vi "Actor Core.vi"(8 "error in":errorcluster, 11 "Data Viewer in":refnum<class "NI Force Task.lvclass">) -> (0 "error out":errorcluster, 3 "Actor out":refnum<class "Actor.lvclass">)   [LabVIEW 2020, in "NI Force Task.lvlib" / "NI Force Task.lvclass"]
doc: "The user interface for this panel.\n----\nCopyright: MGI 2016\nAuthor: Derek Trepanier"
uses:
  NI Force Task.lvclass
  C:/Program Files/National Instruments/LabVIEW 2020/vi.lib/MGI/Panel Manager/Panel Actor/Panel Actor/Panel Actor.lvclass
  C:/Program Files/National Instruments/LabVIEW 2020/vi.lib/ActorFramework/Actor/Actor.lvclass
  <vilib>/ActorFramework/Actor/Actor.lvclass
  Task info df.ctl
  NI Force Task.lvclass/NI Force Task.ctl
  <vilib>/ActorFramework/Actor/Actor.lvclass/Actor.ctl
  <vilib>/ActorFramework/Message Enqueuer/Message Enqueuer.lvclass/Message Enqueuer.ctl
  GUI Interface Messages/MVC Collection Finished Msg/MVC Collection Finished Msg.lvclass/MVC Collection Finished Msg.ctl
  GUI Interface Messages/Force Calibration Finished Msg/Force Calibration Finished Msg.lvclass/Force Calibration Finished Msg.ctl
  GUI Interface Messages/Pot Calibration Finished Msg/Pot Calibration Finished Msg.lvclass/Pot Calibration Finished Msg.ctl
  NI Force Task Messages/Update Template Graph Msg/Update Template Graph Msg.lvclass/Update Template Graph Msg.ctl
  GUI/NI Tasl df.ctl
  Movement Template df.ctl
  <vilib>/Utility/miscctls.llb/LVBoundsTypeDef.ctl
  <vilib>/DAQmx/read.llb/DAQmx Read (Analog 1D Wfm NChan 1Samp).vi
  <vilib>/Analysis/baseanly.llb/Mean (DBL).vi
  <vilib>/ActorFramework/Message Enqueuer/Init from Existing Queue.vi
  <vilib>/ActorFramework/Message Enqueuer/Enqueue.vi
  GUI Interface Messages/MVC Collection Finished Msg/MVC Collection Finished Msg.lvclass
  C:/Program Files/National Instruments/LabVIEW 2020/vi.lib/ActorFramework/Message/Message.lvclass
  GUI Interface Messages/Force Calibration Finished Msg/Force Calibration Finished Msg.lvclass
  GUI Interface Messages/Pot Calibration Finished Msg/Pot Calibration Finished Msg.lvclass
  NI Force Task Messages/Update Template Graph Msg/Update Template Graph Msg.lvclass
  <vilib>/ActorFramework/Stop Msg/Stop Msg.lvclass
  GUI Interface Messages/Task Panel Closed Msg/Task Panel Closed Msg.lvclass
  <vilib>/Waveform/WDTOps.llb/WDT Get Waveform Time Array DBL.vi
  <vilib>/DAQmx/miscellaneous.llb/DAQmx Fill In Error Info.vi
  <vilib>/Analysis/2dsp.llb/Decimate (continuous, DBL).vi
  <vilib>/ActorFramework/Message Priority Queue/Priority Enqueue.vi
  <vilib>/ActorFramework/Message Enqueuer/Message Enqueuer.lvclass
  <vilib>/MGI/Panel Manager/Panel Actor/Panel Actor/Panel Actor.lvclass
  NI Force Task Messages/Process Live Data Q Msg/Process Live Data Q Msg.lvclass
  <vilib>/Analysis/NI_AALBase.lvlib
  <vilib>/Analysis/NI_AALPro.lvlib
  NI Force Task Messages/Process Live Data Q Mov Msg/Process Live Data Q Mov Msg.lvclass
  NI Force Task Messages/Stop Trial Msg/Stop Trial Msg.lvclass
  NI Force Task Messages/End Scanning Trial Msg/End Scanning Trial Msg.lvclass
  NI Force Task Messages/Process Live Data Q EMG Msg/Process Live Data Q EMG Msg.lvclass
panel:
  out "Countdown":string
  in  "EMG Only?":bool
  out "Task Info Backup":T1={"Number of Trials"=1, "Sampling Rate (Hz)"=200, "Trial Duration (s)"=10, "Adjusted MVC (N)"=5.0, "R Phase"=0, "L Phase"=0, "L Pattern"=1, "R Pattern"=1, "Time Between Trials (s)"=5, "Lissajous Speed"=200} {"Lissajous Speed" min=1 max=200; "Time Between Trials (s)" min=1 step=1; "R Pattern" min=1 max=20 step=1; "L Pattern" min=1 max=20 step=1; "L Phase" max=360 step=1; "R Phase" max=360 step=1; "Adjusted MVC (N)" min=1.0 step=1.0; "Trial Duration (s)" min=1 step=1; "Sampling Rate (Hz)" min=1 step=1; "Number of Trials" min=1 step=1}
  in  "Scanning Task?":bool
  in  "Wait":bool
  out "Task Info In":T1={"Number of Trials"=1, "Sampling Rate (Hz)"=200, "Trial Duration (s)"=10, "Adjusted MVC (N)"=5.0, "R Phase"=0, "L Phase"=0, "L Pattern"=1, "R Pattern"=1, "Time Between Trials (s)"=5, "Lissajous Speed"=200} {"Lissajous Speed" min=1 max=200; "Time Between Trials (s)" min=1 step=1; "R Pattern" min=1 max=20 step=1; "L Pattern" min=1 max=20 step=1; "L Phase" max=360 step=1; "R Phase" max=360 step=1; "Adjusted MVC (N)" min=1.0 step=1.0; "Trial Duration (s)" min=1 step=1; "Sampling Rate (Hz)" min=1 step=1; "Number of Trials" min=1 step=1}
  in  "Movement?":bool
  in  "Decimation factor":i32=1
  out "Acquire EMG":bool
  in  "Rate Hz":u16
  out "Live Data":cluster{"Result":dbl[], "Result":dbl[]}(graph)
  in  "Force Calibration Cluster":cluster{"Left":dbl, "Right":dbl}
  in  "Chnl Names":string[](array[string])
  in  "TDMS File Ref":refnum<k34>
  in  "Task Ref":refnum<k21>
  in  "Trial Num":i32
  in  "Stop Acquire":bool
  out "Template Graph":cluster{"Result":dbl[], "Result":dbl[]}(graph)
  # "Right Arm"
  # "Left Arm"
  # "Right Arm"
  # "Left Arm"
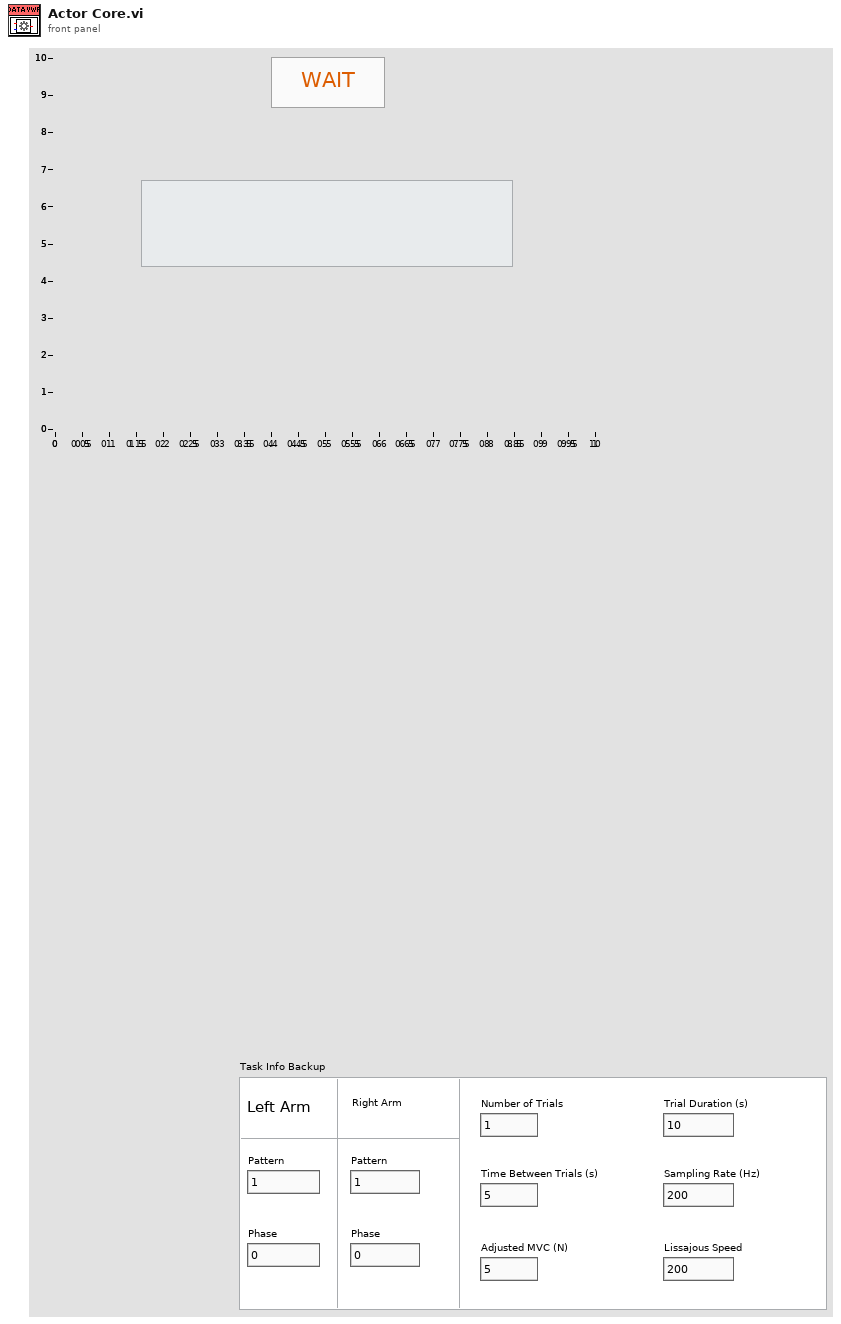
[diagram p1: front panel]
types:
  T1 = typedef "Task info df.ctl" = cluster{"Number of Trials":u8, "Sampling Rate (Hz)":u16, "Trial Duration (s)":u8, "Adjusted MVC (N)":dbl, "R Phase":i32, "L Phase":i32, "L Pattern":u8, "R Pattern":u8, "Time Between Trials (s)":u8, "Lissajous Speed":u16}
  T2 = cluster{"Template Data Update":refnum<user-event>, "Trial Number Update":refnum<user-event>, "Stop Acquire":refnum<user-event>, "Shut Down":refnum<user-event>, "Update Task Plot":refnum<user-event>, "Calibrate Force":refnum<user-event>, "Collect MVC":refnum<user-event>, "Acquire EMG":refnum<user-event>, "Movement? Update":refnum<user-event>, "Calibrate Pot":refnum<user-event>, "Scanning Task?":refnum<user-event>, "EMG only?":refnum<user-event>, "Countdown update":refnum<user-event>}
  T3 = cluster{"Event Registration Refnum":refnum<event-registration>, "Pnl Actor":refnum<event-registration>}
  T4 = typedef "Movement Template df.ctl" = enum16{"Idle", "Update Scanning Template", "Close Helper Loop", "Countdown"}
  T5 = typedef "NI Tasl df.ctl" = enum16{"Idle", "Acquire Force", "Acquire Force and EMG", "Acquire Movement", "Acquire Movement and EMG", "Calibrate Force", "Calibrate Potentiometers", "Collect MVC", "Close Helper Loop", "Collect EMG only", "Countdown"}
  T6 = typedef "LVRectTypeDef.ctl" = cluster{"Left":i16, "Top":i16, "Right":i16, "Bottom":i16}
  T7 = typedef "LVBoundsTypeDef.ctl" = cluster{"Width":u32, "Height":u32}
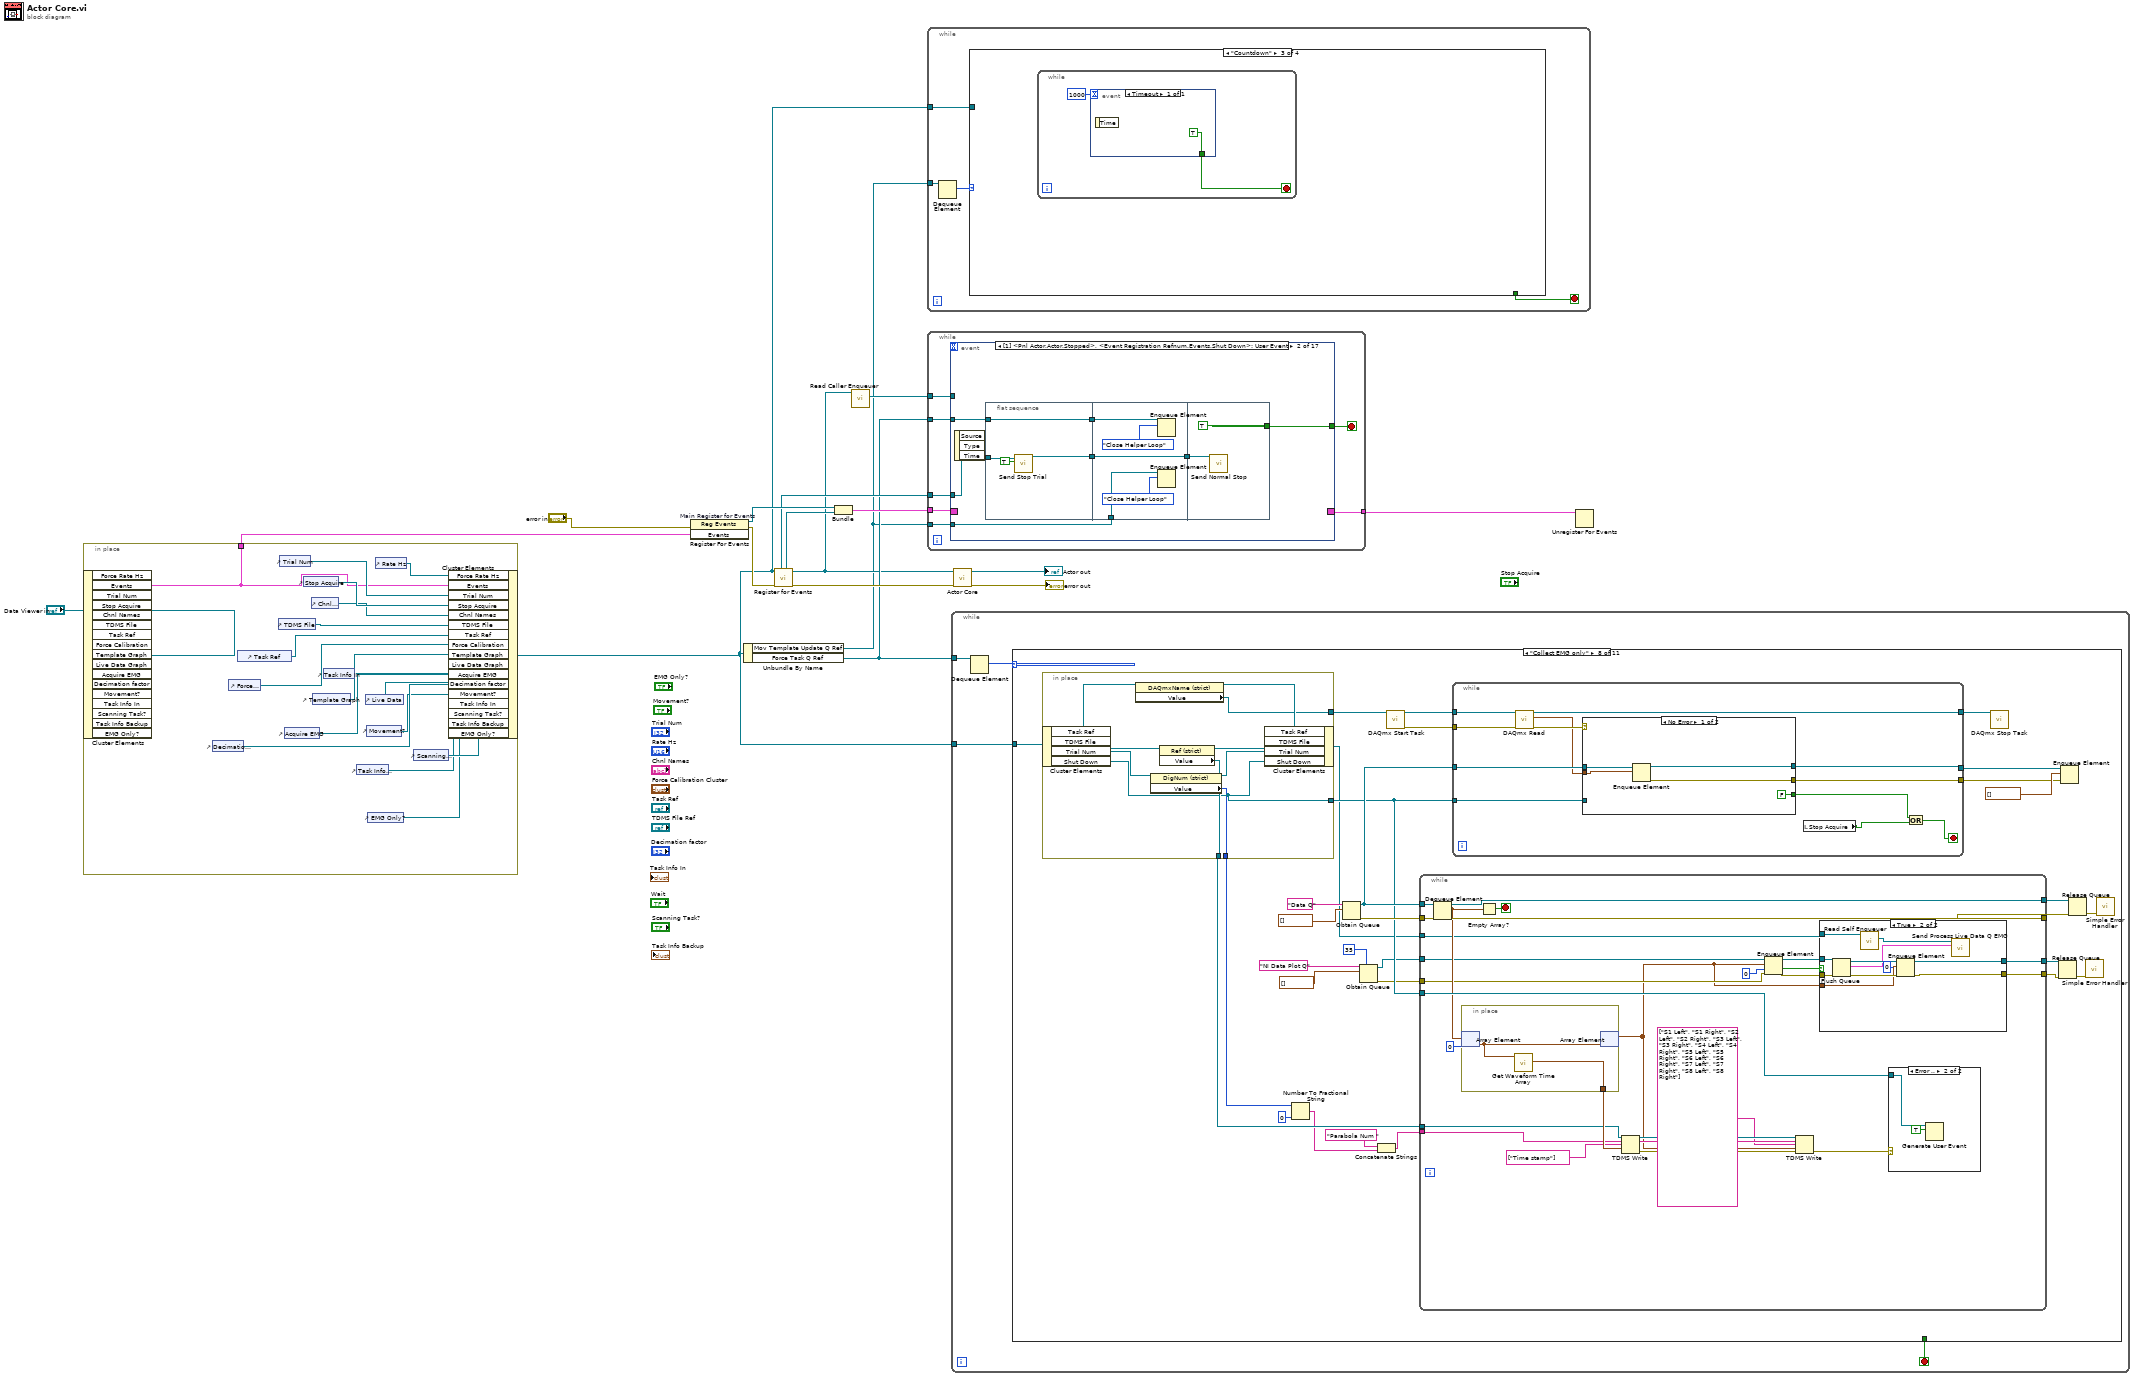
[diagram p0: block diagram]
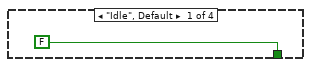
[diagram p2: hidden frame]
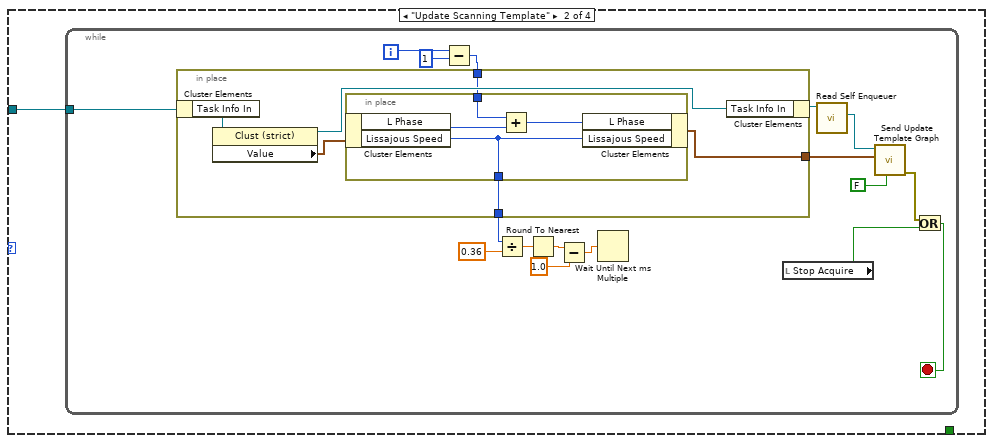
[diagram p3: hidden frame]
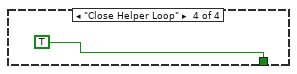
[diagram p4: hidden frame]
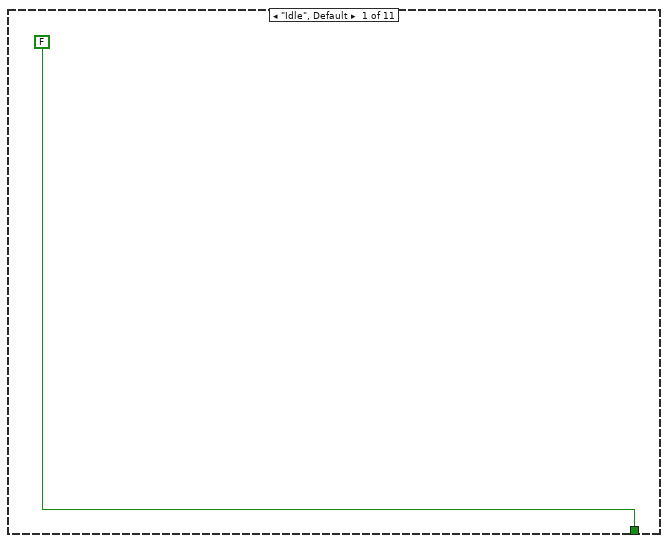
[diagram p5: hidden frame]
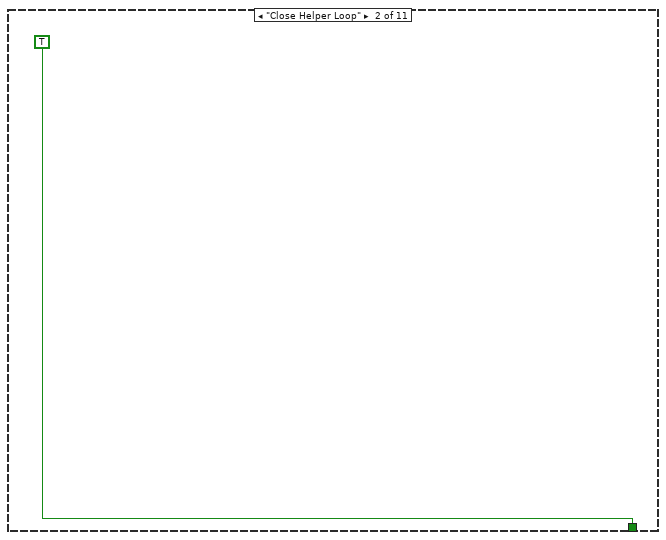
[diagram p6: hidden frame]
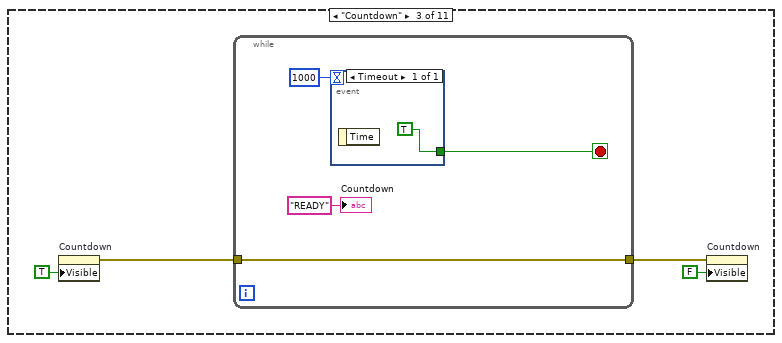
[diagram p7: hidden frame]
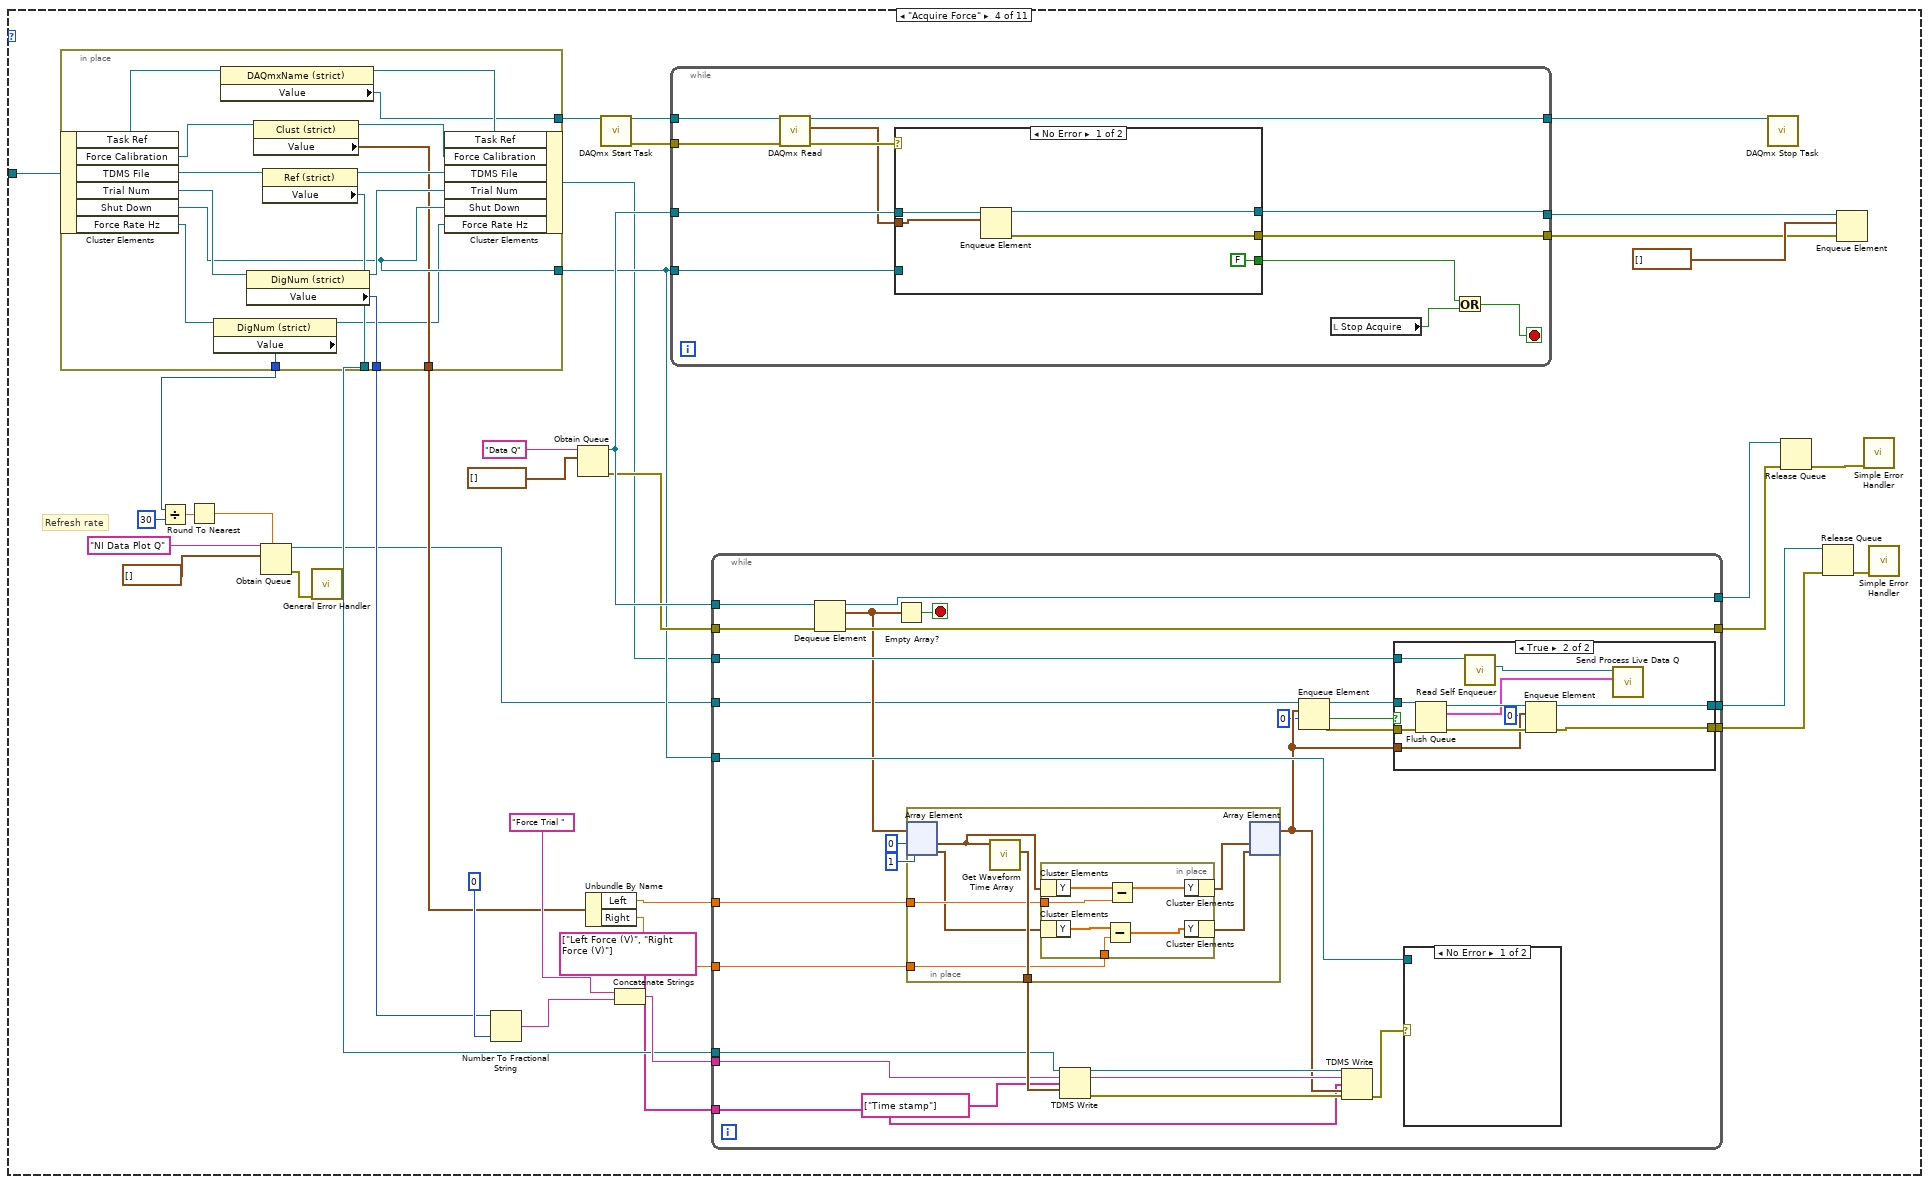
[diagram p8: hidden frame]
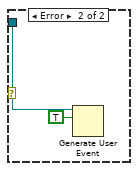
[diagram p10: hidden frame]
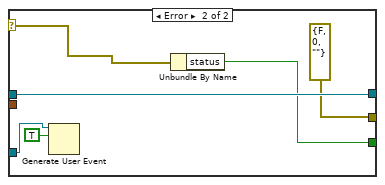
[diagram p11: hidden frame]
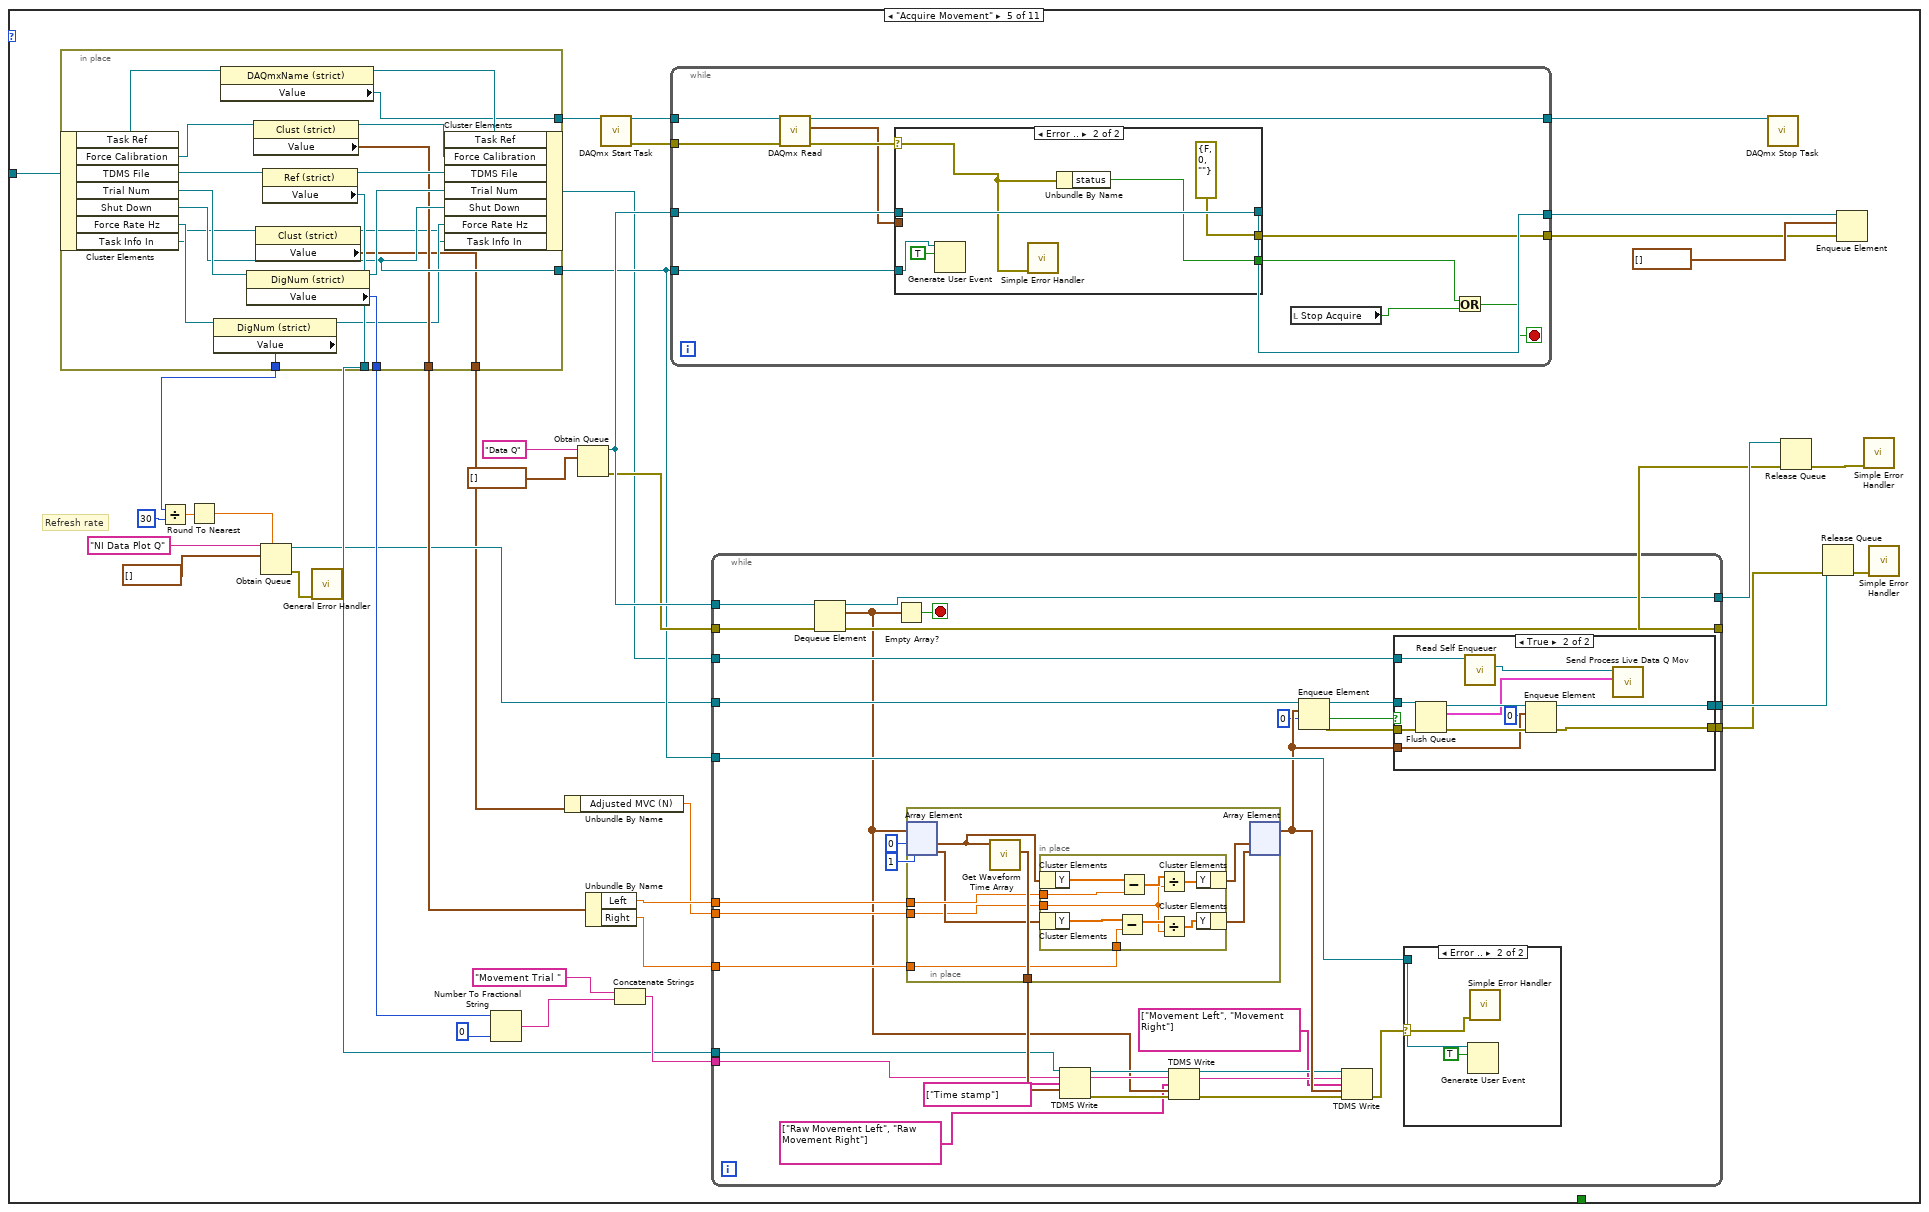
[diagram p12: hidden frame]
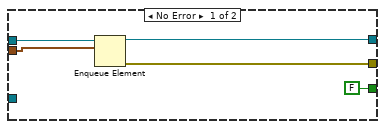
[diagram p15: hidden frame]
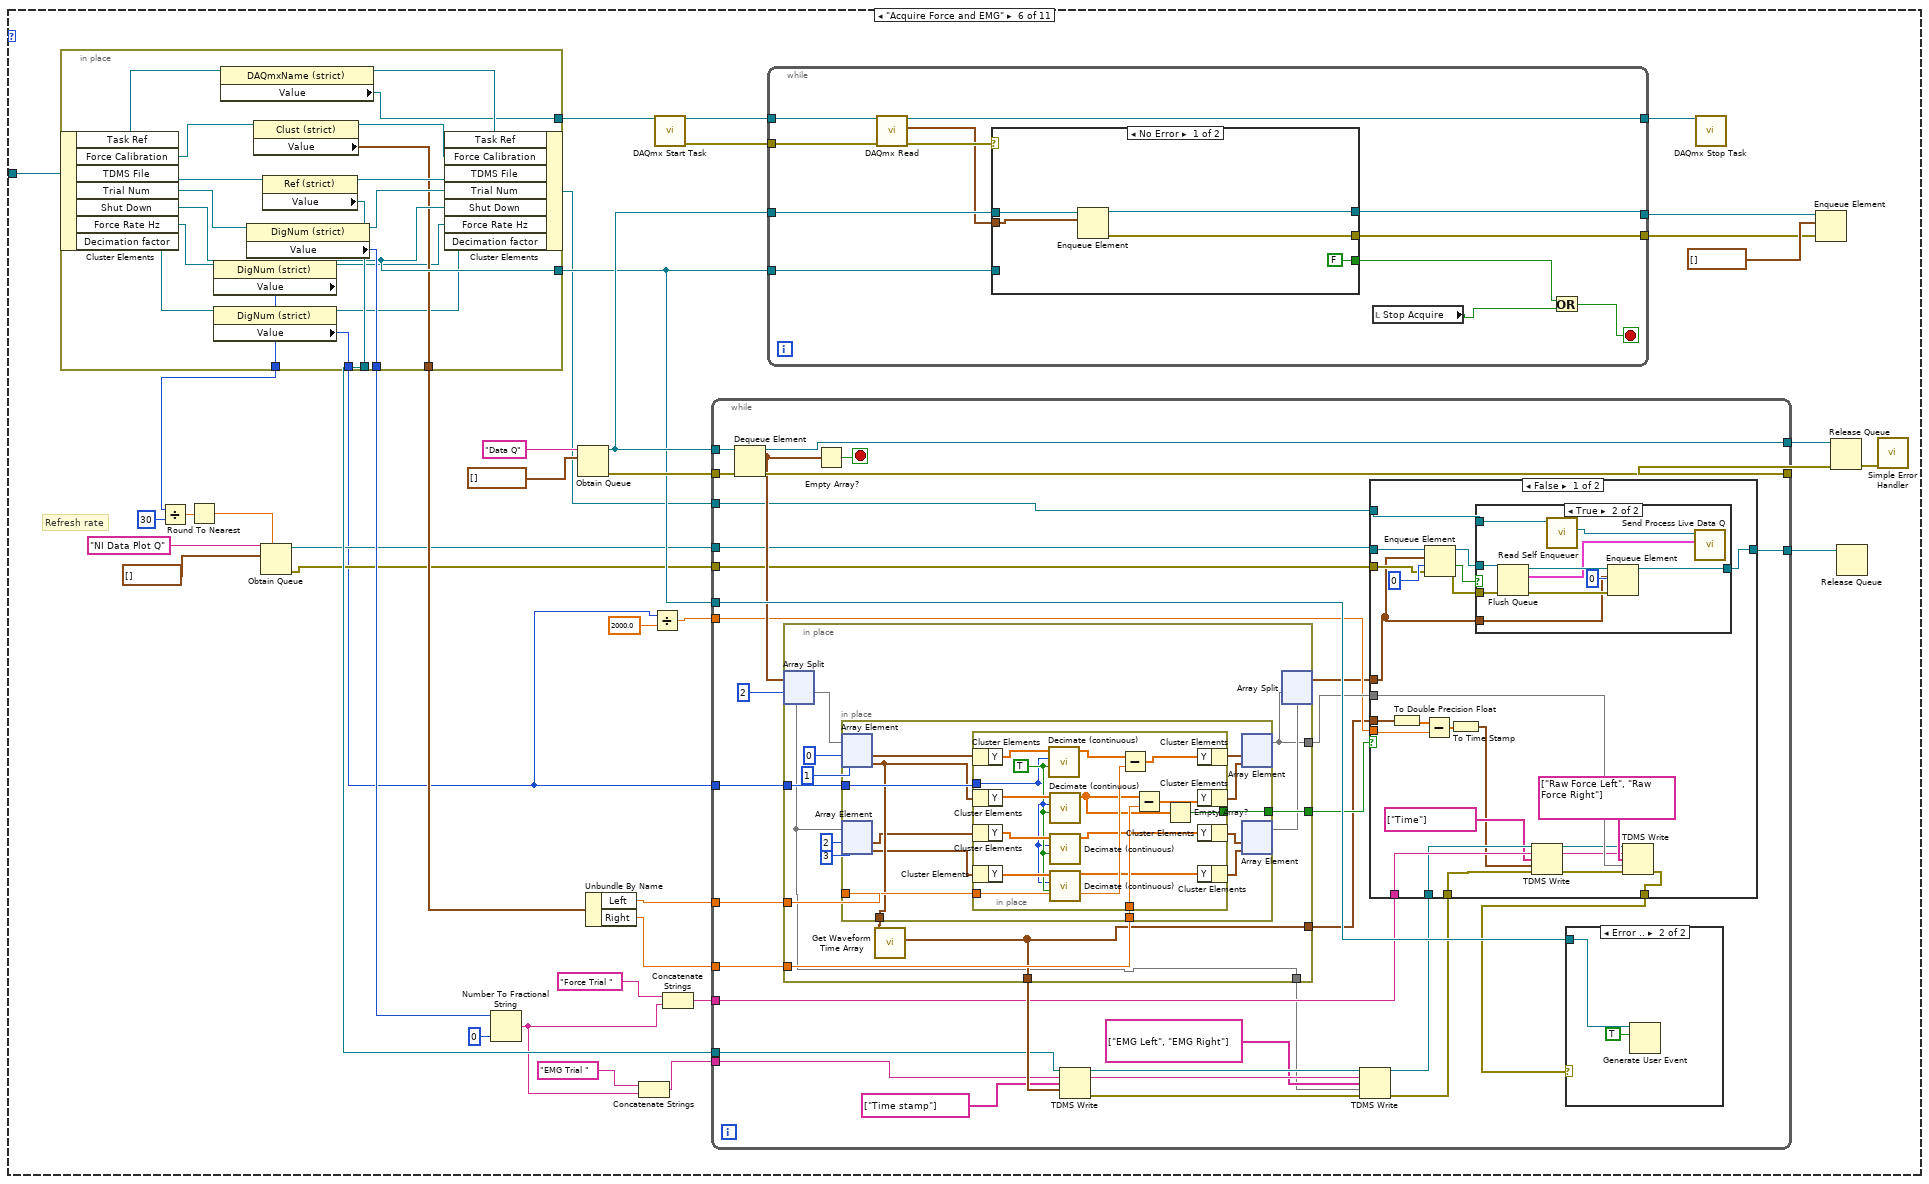
[diagram p16: hidden frame]
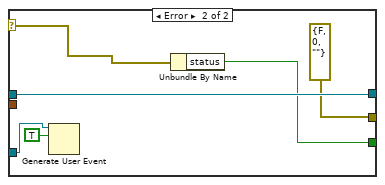
[diagram p20: hidden frame]
diagram:
  n1 = in-place {
    in-place-border: [w28] -> w6
    n2 = in-place-cluster #1("Data Viewer in") -> ("Events"=w28:T2)  [unwired: 16 out]
    n3 = control-ref of="Decimation factor"() -> (w23:refnum<vi>)
    n4 = control-ref of="Force Calibration Cluster"() -> (w29:refnum<vi>)
    n5 = control-ref of="Task Ref"() -> (w31:refnum<vi>)
    n6 = control-ref of="TDMS File"() -> (w30:refnum<vi>)
    n7 = control-ref of="Trial Num"() -> (w34:refnum<vi>)
    n8 = control-ref of="Acquire EMG"() -> (w24:refnum<vi>)
    n9 = control-ref of="Stop Acquire"() -> (w33:refnum<vi>)
    n10 = control-ref of="Chnl Names"() -> (w32:refnum<vi>)
    n11 = control-ref of="Template Graph"() -> (w27:refnum<vi>)
    n12 = control-ref of="Task Info In"() -> (w21:refnum<vi>)
    n13 = control-ref of="Task Info Backup"() -> (w19:refnum<vi>)
    n14 = control-ref of="Live Data"() -> (w26:refnum<vi>)
    n15 = control-ref of="Movement?"() -> (w22:refnum<vi>)
    n16 = control-ref of="EMG Only?"() -> (w18:refnum<vi>)
    n17 = control-ref of="Rate Hz"() -> (w25:refnum<vi>)
    n18 = control-ref of="Scanning Task?"() -> (w20:refnum<vi>)
    n19 = in-place-cluster #1("Force Rate Hz"=w25, "Events"=w28, "Trial Num"=w34, "Stop Acquire"=w33, "Chnl Names"=w32, "TDMS File"=w30, "Task Ref"=w31, "Force Calibration"=w29, "Template Graph"=w27, "Live Data Graph"=w26, "Acquire EMG"=w24, "Decimation factor"=w23, "Movement?"=w22, "Task Info In"=w21, "Scanning Task?"=w20, "Task Info Backup"=w19, "EMG Only?"=w18) -> (w1:refnum<class "NI Force Task.lvclass">)
  }
  n20 = register-events "Main Register for Events"(error in="error in", w6) -> (reference out=w12:refnum<event-registration>, error out=w13:errorcluster)  [unwired: 1 in]
  n21 = Unbundle By Name(w1) -> ("Mov Template Update Q Ref"=w2:refnum<queue>, "Force Task Q Ref"=w5:refnum<queue>)
  n22 = call <vilib>:"Register for Events.vi"("Error In"=w13, "Panel Actor in"=w1) -> ("Error Out"=w15:errorcluster, "Panel Actor out"=w4:refnum<class "NI Force Task.lvclass">, "Pnl Actor"=w11:refnum<event-registration>, "Self Enqueuer"=w7:refnum<class "Message Enqueuer.lvclass">)  [unwired: 6 in]
  n23 = Bundle("Event Registration Refnum"=w12, "Pnl Actor"=w11) -> (w10:T3)  [unwired: 1 in]
  n24 = call <vilib>:"Read Caller Enqueuer.vi"("Actor"=w4) -> ("Caller Enqueuer"=w3:refnum<class "Message Enqueuer.lvclass">)  [unwired: 10 in]
  n25 = while {
    tunnel: w2 -> [w38]
    tunnel: w1 -> [w35]
    stop <- w36 stop-if-true
    n26 = Dequeue Element(queue=w38) -> (element=w37:T4)  [unwired: 2 in, 3 out]
    n27 = case shown="\"Countdown\"" w37 {
      tunnel: [FALSE _ _ TRUE] -> w36
      tunnel: w35 -> [_ w40 _ _]
      frame "Idle", Default {
      }
      frame "Update Scanning Template" {
        n28 = while {
          tunnel: w40 -> [w41]
          i -> [w48]
          stop <- w49 stop-if-true
          n29 = Subtract(x=w48, y=1) -> (x-y=w47:i32)
          n30 = in-place {
            in-place-border: [w60] -> w55
            in-place-border: [w59] -> w52
            in-place-border: w47 -> [w58]
            n31 = in-place-cluster #2(w41) -> ("Task Info In"=w63:refnum<vi>)
            n32 = property class="Clust (strict)"(reference=w63) -> (reference out=w61:refnum<vi>, "Value"=w62:T1)  [unwired: 1 in, 1 out]
            n33 = in-place {
              in-place-border: [w67] -> w60
              in-place-border: w58 -> [w64]
              n34 = in-place-cluster #3(w62) -> ("L Phase"=w66:i32, "Lissajous Speed"=w67:u16)
              n35 = Add(x=w64, y=w66) -> (x+y=w65:i32)
              n36 = in-place-cluster #3("L Phase"=w65, "Lissajous Speed"=w67) -> (w59:T1)
            }
            n37 = in-place-cluster #2("Task Info In"=w61) -> (w54:refnum<class "NI Force Task.lvclass">)
          }
          n38 = Divide(x=w55, y=0.36) -> (x/y=w57:dbl)
          n39 = Round To Nearest(number=w57) -> (nearest integer value=w44:dbl)
          n40 = Subtract(x=w44, y=1.0) -> (x-y=w45:dbl)
          n41 = Wait Until Next ms Multiple(millisecond multiple=w45) -> ()  [unwired: 1 out]
          n42 = local read "Stop Acquire"() -> (w50:bool)
          n43 = call <vilib>:"Read Self Enqueuer.vi"("Actor"=w54) -> ("Self Enqueuer"=w53:refnum<class "Message Enqueuer.lvclass">)  [unwired: 10 in]
          n44 = call "Send Update Template Graph.vi"("Set Task Info?"=FALSE, "Task Info In"=w52, "Message Enqueuer in"=w53) -> ("error out"=w51:errorcluster)  [unwired: 7 in, 1 out]
          n45 = Or(x=w51, y=w50) -> (x .or. y?=w49:bool)
        }
      }
      frame "Countdown" {
        n46 = while {
          stop <- w68 stop-if-true
          n47 = event shown="[0] Timeout" {
            selector: _ -> [_]
            dyn-events: _ -> [_]
            timeout: 1000 -> [_]
            tunnel: [TRUE] -> w68
            event Timeout {
              n48 = event-data() -> ()  [unwired: 1 in, 1 out]
            }
          }
        }
      }
      frame "Close Helper Loop" {
      }
    }
  }
  n49 = while {
    tunnel: w7 -> [w77]
    tunnel: w10 -> [w76]
    tunnel: [w75] -> w9
    tunnel: w5 -> [w74]
    tunnel: w3 -> [w73]
    tunnel: w2 -> [w72]
    stop <- w78 stop-if-true
    n50 = event shown="[1] <Pnl Actor.Actor.Stopped>, <Event Registration Refnum.Events.Shut Down>: User Event" {
      selector: w76 -> [_ _ _ _ _ _ _ _ _ _ _ _ _ _ _ _ _]
      dyn-events: [_ _ _ _ _ _ _ _ _ _ _ _ _ _ _ _ _] -> w75
      timeout: _ -> [_ _ _ _ _ _ _ _ _ _ _ _ _ _ _ _ _]
      tunnel: [_ w84 _ _ _ _ _ _ _ _ _ _ _ _ _ _ _] -> w78
      tunnel: w77 -> [_ w83 _ _ _ _ _ _ _ _ _ _ _ _ _ w166 _]
      tunnel: w74 -> [_ w85 _ _ _ w116 w120 w124 _ w132 _ _ _ _ _ w170 _]
      tunnel: w73 -> [_ _ w97 _ _ _ _ _ _ _ _ _ _ _ _ w167 _]
      tunnel: w72 -> [_ w81 _ _ _ _ _ _ _ w136 _ _ _ _ _ w168 _]
      event Timeout {
        n51 = event-data() -> ()  [unwired: 1 in, 3 out]
      }
      event User Event {
        n52 = event-data() -> ()  [unwired: 1 in, 3 out]
        n53 = flat-sequence {
          tunnel: w85 -> [w89]
          tunnel: [w89] -> w80
          tunnel: w83 -> [w88]
          tunnel: [w86] -> w79
          tunnel: w80 -> [w94]
          tunnel: w79 -> [w92]
          tunnel: [w92] -> w82
          tunnel: w81 -> [w91]
          tunnel: [TRUE] -> w84
          tunnel: w82 -> [w95]
          frame #0 {
            n54 = call "Send Stop Trial.vi"("Stop Acquiring"=TRUE, "Message Enqueuer in"=w88) -> ("Message Enqueuer out"=w86:refnum<class "Message Enqueuer.lvclass">)  [unwired: 8 in, 1 out]
          }
          frame #1 {
            n55 = Enqueue Element(queue=w94, element=NI_Tasl_df."Close Helper Loop") -> ()  [unwired: 2 in, 3 out]
            n56 = Enqueue Element(queue=w91, element=Movement_Template_df."Close Helper Loop") -> ()  [unwired: 2 in, 3 out]
          }
          frame #2 {
            n57 = call <vilib>:"Send Normal Stop.vi"("Message Enqueuer"=w95) -> ()  [unwired: 10 in, 1 out]
          }
        }
      }
      event Panel Close {
        n58 = event-data() -> ()  [unwired: 1 in, 4 out]
        n59 = call "Send Task Panel Closed.vi"("Message Enqueuer"=w97) -> ()  [unwired: 9 in, 2 out]
      }
      event Panel Resize {
        n60 = event-data() -> ("NewBnds"=w100:T6)  [unwired: 1 in]
        n61 = in-place {
          in-place-border: [w106] -> w99
          w102 = i16 50 ("y")
          n62 = in-place-cluster #4(w100) -> ("Right"=w110:i16, "Left"=w109:i16, "Bottom"=w108:i16, "Top"=w107:i16)
          n63 = Subtract(x=w110, y=w109) -> (x-y=w105:i16)
          n64 = Subtract(x=w108, y=w107) -> (x-y=w103:i16)
          n65 = Less Or Equal?(x=w105, y=w103) -> (x <= y?=w111:bool)
          n66 = Subtract(x=w105, y=w102) -> (x-y=w101:i16)
          n67 = Subtract(x=w103, y=w102) -> (x-y=w104:i16)
          n68 = Select(t=w101, s=w111, f=w104) -> (s? t:f=w106:i16)
          n69 = in-place-cluster #4("Right"=w110, "Left"=w109, "Bottom"=w108, "Top"=w107) -> ()  [unwired: 1 out]
        }
        n70 = Bundle(w99, w99) -> (w98:cluster{i16, i16})  [unwired: 1 in]
        n71 = property on="Live Data" class="XYGraph (strict)"("Plot Area Size"=w98) -> ()  [unwired: 2 in, 2 out]
        n72 = property on="Template Graph" class="XYGraph (strict)"("Plot Area Size"=w98) -> ()  [unwired: 2 in, 2 out]
      }
      event User Event {
        n73 = event-data() -> ("X"=w114:dbl[], "Y"=w113:dbl[])  [unwired: 1 in]
        n74 = Bundle("X"=w114, "Y"=w113) -> (→"Template Graph":cluster{"X":dbl[], "Y":dbl[]})  [unwired: 1 in]
      }
      event User Event {
        n75 = event-data() -> ("Calibrate Force"=w115:bool)  [unwired: 1 in, 4 out]
        n76 = case shown="True" w115 {
          tunnel: w116 -> [_ w118]
          frame False {
          }
          frame True {
            n77 = Enqueue Element(queue=w118, element=NI_Tasl_df."Calibrate Force") -> ()  [unwired: 2 in, 3 out]
          }
        }
      }
      event User Event {
        n78 = event-data() -> ("Calibrate Pot"=w119:bool)  [unwired: 1 in]
        n79 = case shown="True" w119 {
          tunnel: w120 -> [_ w122]
          frame False {
          }
          frame True {
            n80 = Enqueue Element(queue=w122, element=NI_Tasl_df."Calibrate Potentiometers") -> ()  [unwired: 2 in, 3 out]
          }
        }
      }
      event User Event {
        n81 = event-data() -> ("Collect MVC"=w123:bool)  [unwired: 1 in, 4 out]
        n82 = case shown="True" w123 {
          tunnel: w124 -> [_ w126]
          frame False {
          }
          frame True {
            n83 = Enqueue Element(queue=w126, element=NI_Tasl_df."Collect MVC") -> ()  [unwired: 2 in, 3 out]
          }
        }
      }
      event User Event {
        n84 = event-data() -> ("X Data"=w129:dbl[], "Y Data"=w128:dbl[])  [unwired: 1 in]
        n85 = Bundle("X Data"=w129, "Y Data"=w128) -> (→"Live Data":cluster{"X Data":dbl[], "Y Data":dbl[]})  [unwired: 1 in]
      }
      event User Event {
        n86 = event-data() -> ()  [unwired: 1 in, 1 out]
        n87 = property on="Wait" class="Bool (strict)"("Visible"=FALSE) -> ()  [unwired: 2 in, 2 out]
        n88 = Enqueue Element(queue=w132, element=NI_Tasl_df."Countdown") -> (queue out=w133:refnum<queue>, error out=w130:errorcluster)  [unwired: 2 in, 1 out]
        n89 = local read "EMG Only?"() -> (w134:bool)
        n90 = case shown="False" w134 {
          tunnel: w136 -> [w141 _]
          tunnel: w133 -> [w137 w161]
          tunnel: w130 -> [_ w159]
          frame False {
            n91 = local read "Scanning Task?"() -> (w139:bool)
            n92 = local read "Acquire EMG"() -> (w140:bool)
            n93 = local read "Movement?"() -> (w138:bool)
            n94 = case shown="True" w139 {
              tunnel: w141 -> [_ w158]
              frame False {
              }
              frame True {
                n95 = Enqueue Element(queue=w158, element=Movement_Template_df."Countdown") -> (queue out=w156:refnum<queue>, error out=w155:errorcluster)  [unwired: 2 in, 1 out]
                n96 = Enqueue Element(queue=w156, element=Movement_Template_df."Update Scanning Template", error in (no error)=w155) -> ()  [unwired: 1 in, 3 out]
              }
            }
            n97 = case shown="True" w138 {
              tunnel: w140 -> [w142 w149]
              tunnel: w137 -> [w143 w148]
              frame False {
                n98 = case shown="False" w142 {
                  tunnel: w143 -> [w145 w146]
                  frame False {
                    n99 = Enqueue Element(queue=w145, element=NI_Tasl_df."Acquire Force") -> ()  [unwired: 2 in, 3 out]
                  }
                  frame True {
                    n100 = Enqueue Element(queue=w146, element=NI_Tasl_df."Acquire Force and EMG") -> ()  [unwired: 2 in, 3 out]
                  }
                }
              }
              frame True {
                n101 = case shown="True" w149 {
                  tunnel: w148 -> [w150 w152]
                  frame False {
                    n102 = Enqueue Element(queue=w150, element=NI_Tasl_df."Acquire Movement") -> ()  [unwired: 2 in, 3 out]
                  }
                  frame True {
                    n103 = Enqueue Element(queue=w152, element=NI_Tasl_df."Acquire Movement and EMG") -> ()  [unwired: 2 in, 3 out]
                  }
                }
              }
            }
          }
          frame True {
            n104 = Enqueue Element(queue=w161, element=NI_Tasl_df."Collect EMG only", error in (no error)=w159) -> ()  [unwired: 1 in, 3 out]
          }
        }
      }
      event User Event {
        n105 = event-data() -> ()  [unwired: 1 in, 1 out]
      }
      event User Event {
        n106 = event-data() -> ("EMG only?"=w162:bool)  [unwired: 1 in]
        n107 = property on="EMG Only?" class="Bool (strict)"("Val(Sgnl)"=w162) -> ()  [unwired: 2 in, 2 out]
      }
      event User Event {
        n108 = event-data() -> ("Scanning?"=w163:bool)  [unwired: 1 in]
        n109 = property on="Scanning Task?" class="Bool (strict)"("Val(Sgnl)"=w163) -> ()  [unwired: 2 in, 2 out]
      }
      event User Event {
        n110 = event-data() -> ("Movement?"=w164:bool)  [unwired: 1 in]
        n111 = property on="Movement?" class="Bool (strict)"("Val(Sgnl)"=w164) -> ()  [unwired: 2 in, 2 out]
      }
      event User Event {
        n112 = event-data() -> ("Acquire EMG"=→"Acquire EMG":bool)  [unwired: 1 in]
      }
      event User Event {
        n113 = event-data() -> ("Stop Acquire"=w169:bool)  [unwired: 1 in]
        n114 = property on="Stop Acquire" class="Bool (strict)"("Val(Sgnl)"=w169) -> ()  [unwired: 2 in, 2 out]
        n115 = case shown="True" w169 {
          tunnel: w170 -> [_ w180]
          tunnel: w168 -> [_ w178]
          tunnel: w167 -> [_ _]
          tunnel: w166 -> [_ w174]
          frame False {
          }
          frame True {
            n116 = Enqueue Element(queue=w180, element=NI_Tasl_df."Idle") -> (error out=w176:errorcluster)  [unwired: 2 in, 2 out]
            n117 = Enqueue Element(queue=w178, element=Movement_Template_df."Idle") -> (error out=w172:errorcluster)  [unwired: 2 in, 2 out]
            n118 = property on="Wait" class="Bool (strict)"(error in=w176, "Visible"=TRUE) -> (error out=w173:errorcluster)  [unwired: 1 in, 1 out]
            n119 = Merge Errors(w173, w172) -> (w171:errorcluster)
            n120 = call "Send End Scanning Trial.vi"("error in (no error)"=w171, "Message Enqueuer in"=w174) -> ()  [unwired: 8 in, 2 out]
          }
        }
      }
      event User Event {
        n121 = event-data() -> ()  [unwired: 1 in, 1 out]
        n122 = case shown="True" TRUE {
          frame False {
          }
          frame True {
            w182 = T7 {"Width"=550, "Height"=550} ("Plot Area:Size")
            n123 = property on="Template Graph" class="XYGraph (strict)"("Plot Area Size"=w182) -> ()  [unwired: 2 in, 2 out]
            n124 = property on="Live Data" class="XYGraph (strict)"("Plot Area Size"=w182) -> ()  [unwired: 2 in, 2 out]
          }
        }
      }
    }
  }
  n125 = while {
    tunnel: w5 -> [w185]
    tunnel: w1 -> [w184]
    stop <- w186 stop-if-true
    n126 = Dequeue Element(queue=w185) -> (element=w183:T5)  [unwired: 2 in, 3 out]
    n127 = case shown="\"Collect EMG only\"" w183 {
      tunnel: [FALSE TRUE _ _ _ _ _ _ _ _ _] -> w186
      tunnel: w184 -> [_ _ _ w218 w353 w503 w700 w908 w1027 w1140 w1211]
      frame "Idle", Default {
      }
      frame "Close Helper Loop" {
      }
      frame "Countdown" {
        n128 = property on="Countdown" class="Str"("Visible"=TRUE) -> (error out=w191:errorcluster)  [unwired: 2 in, 1 out]
        n129 = while {
          tunnel: w191 -> [w195]
          tunnel: [w195] -> w190
          stop <- w194 stop-if-true
          n130 = event shown="[0] Timeout" {
            selector: _ -> [_]
            dyn-events: _ -> [_]
            timeout: 1000 -> [_]
            tunnel: [TRUE] -> w194
            event Timeout {
              n131 = event-data() -> ()  [unwired: 1 in, 1 out]
            }
          }
          "Countdown" <- "READY" ("Countdown")
        }
        n132 = property on="Countdown" class="Str"(error in=w190, "Visible"=FALSE) -> ()  [unwired: 1 in, 2 out]
      }
      frame "Acquire Force" {
        # "Refresh rate"
        n133 = in-place {
          in-place-border: [w245] -> w217
          in-place-border: [w244] -> w216
          in-place-border: [w241] -> w215
          in-place-border: [w240] -> w214
          in-place-border: [w239] -> w213
          in-place-border: [w238] -> w204
          n134 = in-place-cluster #5(w218) -> ("Task Ref"=w251:refnum<vi>, "Force Calibration"=w249:refnum<vi>, "TDMS File"=w246:refnum<vi>, "Trial Num"=w243:refnum<vi>, "Shut Down"=w240:refnum<user-event>, "Force Rate Hz"=w237:refnum<vi>)
          n135 = property class="DigNum (strict)"(reference=w237) -> (reference out=w236:refnum<vi>, "Value"=w238:u16)  [unwired: 1 in, 1 out]
          n136 = property class="DAQmxName (strict)"(reference=w251) -> (reference out=w250:refnum<vi>, "Value"=w245:refnum<k21>)  [unwired: 1 in, 1 out]
          n137 = property class="DigNum (strict)"(reference=w243) -> (reference out=w242:refnum<vi>, "Value"=w241:i32)  [unwired: 1 in, 1 out]
          n138 = property class="Clust (strict)"(reference=w249) -> (reference out=w248:refnum<vi>, "Value"=w239:cluster{"Left":dbl, "Right":dbl})  [unwired: 1 in, 1 out]
          n139 = property class="Ref (strict)"(reference=w246) -> (reference out=w247:refnum<vi>, "Value"=w244:refnum<k34>)  [unwired: 1 in, 1 out]
          n140 = in-place-cluster #5("Task Ref"=w250, "Force Calibration"=w248, "TDMS File"=w247, "Trial Num"=w242, "Shut Down"=w240, "Force Rate Hz"=w236) -> (w210:refnum<class "NI Force Task.lvclass">)
        }
        n141 = Divide(x=w204, y=u16 30) -> (x/y=w206:dbl)
        n142 = Round To Nearest(number=w206) -> (nearest integer value=w199:dbl)
        n143 = Obtain Queue(max queue size (-1, unlimited)=w199, name (unnamed)="NI Data Plot Q", element data type=waveform(dbl)[] [] ("data")) -> (queue out=w201:refnum<queue>, error out=w200:errorcluster)  [unwired: 2 in, 1 out]
        n144 = call <vilib>:"General Error Handler.vi"("error in (no error)"=w200) -> ()  [unwired: 10 in, 5 out]
        n145 = Number To Fractional String(number=w215, precision (6)=i16 0) -> (F-format string=w227:string)  [unwired: 2 in]
        n146 = Obtain Queue(name (unnamed)="Data Q", element data type=waveform(dbl)[] [] ("data")) -> (queue out=w231:refnum<queue>, error out=w221:errorcluster)  [unwired: 3 in, 1 out]
        n147 = Unbundle By Name(w213) -> ("Left"=w212:dbl, "Right"=w211:dbl)
        n148 = call <vilib>:"DAQmx Start Task.vi"("task/channels in"=w217) -> ("task out"=w235:refnum<k21>, "error out"=w234:errorcluster)  [unwired: 13 in]
        n149 = Concatenate Strings("Force Trial " ("string"), w227) -> (w224:string)
        n150 = while {
          tunnel: w235 -> [w320]
          tunnel: w234 -> [w319]
          tunnel: w231 -> [w317]
          tunnel: [w316] -> w228
          tunnel: [w314] -> w230
          tunnel: [w311] -> w219
          tunnel: w214 -> [w310]
          stop <- w313 stop-if-true
          n151 = call-poly <vilib>:"DAQmx Read.vi"("task/channels in"=w320, "error in"=w319) -> ("task out"=w316:refnum<k21>, "data"=w315:waveform(dbl)[], "error out"=w318:errorcluster)  [unwired: 11 in]
          n152 = case shown="No Error" w318 {
            selector: w318 -> [_ w328]
            tunnel: w317 -> [w325 w331]
            tunnel: w315 -> [w324 _]
            tunnel: [w323 w331] -> w314
            tunnel: [FALSE ("x") w329] -> w312
            tunnel: [w321 errorcluster {"status"=FALSE, "code"=0, "source"=""} ("error out")] -> w311
            tunnel: w310 -> [_ w326]
            frame No Error {
              n153 = Enqueue Element(queue=w325, element=w324) -> (queue out=w323:refnum<queue>, error out=w321:errorcluster)  [unwired: 2 in, 1 out]
            }
            frame Error {
              n154 = Generate User Event(user event=w326, event data cluster=TRUE ("event data")) -> ()  [unwired: 2 in, 2 out]
              n155 = Unbundle By Name(w328) -> ("status"=w329:bool)
            }
          }
          n156 = local read "Stop Acquire"() -> (w309:bool)
          n157 = Or(x=w312, y=w309) -> (x .or. y?=w313:bool)
        }
        n158 = while {
          tunnel: w231 -> [w275]
          tunnel: w224 -> [w273]
          tunnel: [w272] -> w222
          tunnel: w221 -> [w271]
          tunnel: [w270] -> w220
          tunnel: w216 -> [w267]
          tunnel: w214 -> [w266]
          tunnel: w212 -> [w265]
          tunnel: w211 -> [w264]
          tunnel: w210 -> [w262]
          tunnel: [w257] -> w209
          tunnel: [w256] -> w207
          tunnel: w201 -> [w255]
          tunnel: string[] ["Left Force (V)", "Right Force (V)"] ("Chnl Names") -> [w252]
          stop <- w274 stop-if-true
          n159 = Dequeue Element(queue=w275, error in (no error)=w271) -> (queue out=w272:refnum<queue>, element=w259:waveform(dbl)[], error out=w270:errorcluster)  [unwired: 1 in, 1 out]
          n160 = Empty Array?(array=w259) -> (empty?=w274:bool)
          n161 = in-place {
            in-place-border: [w302] -> w279
            in-place-border: w265 -> [w299]
            in-place-border: w264 -> [w298]
            n162 = in-place-array #6(w259, 0, 1) -> (w301:waveform(dbl), w297:waveform(dbl))
            n163 = call-poly <vilib>:"Get Waveform Time Array.vi"("waveform in"=w301) -> ("X array"=w302:timestamp[])  [unwired: 9 in, 1 out]
            n164 = in-place {
              in-place-border: w299 -> [w305]
              in-place-border: w298 -> [w304]
              n165 = in-place-cluster #7(w301) -> ("Y"=w308:dbl[])
              n166 = in-place-cluster #8(w297) -> ("Y"=w306:dbl[])
              n167 = Subtract(x=w306, y=w304) -> (x-y=w303:dbl[])
              n168 = Subtract(x=w308, y=w305) -> (x-y=w307:dbl[])
              n169 = in-place-cluster #7("Y"=w307) -> (w300:waveform(dbl))
              n170 = in-place-cluster #8("Y"=w303) -> (w296:waveform(dbl))
            }
            n171 = in-place-array #6(w300, w296) -> (w258:waveform(dbl)[])  [unwired: 2 out]
          }
          n172 = TDMS Write(0:w267, 5:w273, 7:string[] ["Time stamp"] ("channel name(s) in (Untitled)"), 9:w279) -> (4:w277:refnum<k34>, 6:w276:string, 15:w269:errorcluster)  [unwired: 2 in, 1 out]
          n173 = Enqueue Element(queue=w255, element=w258, timeout in ms (-1)=0) -> (queue out=w261:refnum<queue>, timed out?=w263:bool, error out=w260:errorcluster)  [unwired: 1 in]
          n174 = TDMS Write(0:w277, 5:w276, 7:w252, 9:w258, 11:w269) -> (15:w268:errorcluster)  [unwired: 1 in, 3 out]
          n175 = case shown="True" w263 {
            tunnel: w262 -> [_ w291]
            tunnel: w261 -> [w282 w290]
            tunnel: w260 -> [w281 w289]
            tunnel: w258 -> [_ w288]
            tunnel: [w282 w285] -> w257
            tunnel: [w281 w284] -> w256
            frame False {
            }
            frame True {
              n176 = Flush Queue(queue=w290, error in (no error)=w289) -> (queue out=w293:refnum<queue>, remaining elements=w286:cluster{"data":waveform(dbl)[]}[], error out=w292:errorcluster)
              n177 = call <vilib>:"Read Self Enqueuer.vi"("Actor"=w291) -> ("Self Enqueuer"=w287:refnum<class "Message Enqueuer.lvclass">)  [unwired: 10 in]
              n178 = Enqueue Element(queue=w293, element=w288, timeout in ms (-1)=0, error in (no error)=w292) -> (queue out=w285:refnum<queue>, error out=w284:errorcluster)  [unwired: 1 out]
              n179 = call "Send Process Live Data Q.vi"("Live Data Q Elements"=w286, "Message Enqueuer in"=w287) -> ()  [unwired: 8 in, 2 out]
            }
          }
          n180 = case shown="No Error" w268 {
            tunnel: w266 -> [_ w294]
            frame No Error {
            }
            frame Error {
              n181 = Generate User Event(user event=w294, event data cluster=TRUE ("event data")) -> ()  [unwired: 2 in, 2 out]
            }
          }
        }
        n182 = call <vilib>:"DAQmx Stop Task.vi"("task/channels in"=w228) -> ()  [unwired: 13 in, 2 out]
        n183 = Release Queue(queue=w222, error in (no error)=w220) -> (error out=w223:errorcluster)  [unwired: 1 in, 2 out]
        n184 = Release Queue(queue=w209, error in (no error)=w207) -> (error out=w208:errorcluster)  [unwired: 1 in, 2 out]
        n185 = Enqueue Element(queue=w230, element=waveform(dbl)[] [] ("data"), error in (no error)=w219) -> ()  [unwired: 1 in, 3 out]
        n186 = call <vilib>:"Simple Error Handler.vi"("error in (no error)"=w223) -> ()  [unwired: 4 in, 5 out]
        n187 = call <vilib>:"Simple Error Handler.vi"("error in (no error)"=w208) -> ()  [unwired: 4 in, 5 out]
      }
      frame "Acquire Movement" {
        # "Refresh rate"
        n188 = in-place {
          in-place-border: [w383] -> w352
          in-place-border: [w382] -> w351
          in-place-border: [w379] -> w350
          in-place-border: [w378] -> w349
          in-place-border: [w377] -> w348
          in-place-border: [w376] -> w339
          in-place-border: [w371] -> w333
          n189 = in-place-cluster #9(w353) -> ("Task Ref"=w389:refnum<vi>, "Force Calibration"=w387:refnum<vi>, "TDMS File"=w384:refnum<vi>, "Trial Num"=w381:refnum<vi>, "Shut Down"=w378:refnum<user-event>, "Force Rate Hz"=w375:refnum<vi>, "Task Info In"=w373:refnum<vi>)
          n190 = property class="DigNum (strict)"(reference=w375) -> (reference out=w374:refnum<vi>, "Value"=w376:u16)  [unwired: 1 in, 1 out]
          n191 = property class="DAQmxName (strict)"(reference=w389) -> (reference out=w388:refnum<vi>, "Value"=w383:refnum<k21>)  [unwired: 1 in, 1 out]
          n192 = property class="DigNum (strict)"(reference=w381) -> (reference out=w380:refnum<vi>, "Value"=w379:i32)  [unwired: 1 in, 1 out]
          n193 = property class="Clust (strict)"(reference=w387) -> (reference out=w386:refnum<vi>, "Value"=w377:cluster{"Left":dbl, "Right":dbl})  [unwired: 1 in, 1 out]
          n194 = property class="Clust (strict)"(reference=w373) -> (reference out=w372:refnum<vi>, "Value"=w371:T1)  [unwired: 1 in, 1 out]
          n195 = property class="Ref (strict)"(reference=w384) -> (reference out=w385:refnum<vi>, "Value"=w382:refnum<k34>)  [unwired: 1 in, 1 out]
          n196 = in-place-cluster #9("Task Ref"=w388, "Force Calibration"=w386, "TDMS File"=w385, "Trial Num"=w380, "Shut Down"=w378, "Force Rate Hz"=w374, "Task Info In"=w372) -> (w345:refnum<class "NI Force Task.lvclass">)
        }
        n197 = Divide(x=w339, y=u16 30) -> (x/y=w341:dbl)
        n198 = Round To Nearest(number=w341) -> (nearest integer value=w334:dbl)
        n199 = Obtain Queue(max queue size (-1, unlimited)=w334, name (unnamed)="NI Data Plot Q", element data type=waveform(dbl)[] [] ("data")) -> (queue out=w336:refnum<queue>, error out=w335:errorcluster)  [unwired: 2 in, 1 out]
        n200 = call <vilib>:"General Error Handler.vi"("error in (no error)"=w335) -> ()  [unwired: 10 in, 5 out]
        n201 = Number To Fractional String(number=w350, precision (6)=i16 0) -> (F-format string=w362:string)  [unwired: 2 in]
        n202 = Unbundle By Name(w333) -> ("Adjusted MVC (N)"=w332:dbl)
        n203 = Obtain Queue(name (unnamed)="Data Q", element data type=waveform(dbl)[] [] ("data")) -> (queue out=w366:refnum<queue>, error out=w356:errorcluster)  [unwired: 3 in, 1 out]
        n204 = Unbundle By Name(w348) -> ("Left"=w347:dbl, "Right"=w346:dbl)
        n205 = call <vilib>:"DAQmx Start Task.vi"("task/channels in"=w352) -> ("task out"=w370:refnum<k21>, "error out"=w369:errorcluster)  [unwired: 13 in]
        n206 = Concatenate Strings("Movement Trial " ("string"), w362) -> (w359:string)
        n207 = while {
          tunnel: w370 -> [w468]
          tunnel: w369 -> [w467]
          tunnel: w366 -> [w465]
          tunnel: [w464] -> w363
          tunnel: [w462] -> w365
          tunnel: [w459] -> w354
          tunnel: w349 -> [w458]
          stop <- w461 stop-if-true
          n208 = call-poly <vilib>:"DAQmx Read.vi"("task/channels in"=w468, "error in"=w467) -> ("task out"=w464:refnum<k21>, "data"=w463:waveform(dbl)[], "error out"=w466:errorcluster)  [unwired: 11 in]
          n209 = case shown="Error .." w466 {
            selector: w466 -> [_ w474]
            tunnel: w465 -> [w473 w479]
            tunnel: w463 -> [w472 _]
            tunnel: [w471 w479] -> w462
            tunnel: [FALSE ("x") w477] -> w460
            tunnel: [w469 errorcluster {"status"=FALSE, "code"=0, "source"=""} ("error out")] -> w459
            tunnel: w458 -> [_ w475]
            frame No Error {
              n210 = Enqueue Element(queue=w473, element=w472) -> (queue out=w471:refnum<queue>, error out=w469:errorcluster)  [unwired: 2 in, 1 out]
            }
            frame Error {
              n211 = Generate User Event(user event=w475, event data cluster=TRUE ("event data")) -> ()  [unwired: 2 in, 2 out]
              n212 = call <vilib>:"Simple Error Handler.vi"("error in (no error)"=w474) -> ()  [unwired: 4 in, 5 out]
              n213 = Unbundle By Name(w474) -> ("status"=w477:bool)
            }
          }
          n214 = local read "Stop Acquire"() -> (w457:bool)
          n215 = Or(x=w460, y=w457) -> (x .or. y?=w461:bool)
        }
        n216 = while {
          tunnel: w366 -> [w420]
          tunnel: w359 -> [w418]
          tunnel: [w417] -> w357
          tunnel: w356 -> [w416]
          tunnel: [w415] -> w355
          tunnel: w351 -> [w413]
          tunnel: w349 -> [w412]
          tunnel: w347 -> [w411]
          tunnel: w346 -> [w410]
          tunnel: w345 -> [w408]
          tunnel: [w404] -> w344
          tunnel: [w403] -> w342
          tunnel: w336 -> [w402]
          tunnel: w332 -> [w399]
          stop <- w419 stop-if-true
          n217 = Dequeue Element(queue=w420, error in (no error)=w416) -> (queue out=w417:refnum<queue>, element=w392:waveform(dbl)[], error out=w415:errorcluster)  [unwired: 1 in, 1 out]
          n218 = Empty Array?(array=w392) -> (empty?=w419:bool)
          n219 = in-place {
            in-place-border: [w447] -> w422
            in-place-border: w411 -> [w444]
            in-place-border: w410 -> [w443]
            in-place-border: w399 -> [w440]
            n220 = in-place-array #10(w392, 0, 1) -> (w446:waveform(dbl), w442:waveform(dbl))
            n221 = call-poly <vilib>:"Get Waveform Time Array.vi"("waveform in"=w446) -> ("X array"=w447:timestamp[])  [unwired: 9 in, 1 out]
            n222 = in-place {
              in-place-border: w444 -> [w454]
              in-place-border: w443 -> [w453]
              in-place-border: w440 -> [w448]
              n223 = in-place-cluster #11(w446) -> ("Y"=w456:dbl[])
              n224 = in-place-cluster #12(w442) -> ("Y"=w455:dbl[])
              n225 = Subtract(x=w455, y=w453) -> (x-y=w449:dbl[])
              n226 = Subtract(x=w456, y=w454) -> (x-y=w452:dbl[])
              n227 = Divide(x=w452, y=w448) -> (x/y=w450:dbl[])
              n228 = Divide(x=w449, y=w448) -> (x/y=w451:dbl[])
              n229 = in-place-cluster #11("Y"=w450) -> (w445:waveform(dbl))
              n230 = in-place-cluster #12("Y"=w451) -> (w441:waveform(dbl))
            }
            n231 = in-place-array #10(w445, w441) -> (w405:waveform(dbl)[])  [unwired: 2 out]
          }
          n232 = TDMS Write(0:w413, 5:w418, 7:string[] ["Time stamp"] ("channel name(s) in (Untitled)"), 9:w422) -> (4:w397:refnum<k34>, 6:w398:string, 15:w394:errorcluster)  [unwired: 2 in, 1 out]
          n233 = TDMS Write(0:w397, 5:w398, 7:string[] ["Raw Movement Left", "Raw Movement Right"] ("Chnl Names"), 9:w392, 11:w394) -> (4:w396:refnum<k34>, 6:w395:string, 15:w393:errorcluster)  [unwired: 1 in, 1 out]
          n234 = Enqueue Element(queue=w402, element=w405, timeout in ms (-1)=0) -> (queue out=w407:refnum<queue>, timed out?=w409:bool, error out=w406:errorcluster)  [unwired: 1 in]
          n235 = TDMS Write(0:w396, 5:w395, 7:string[] ["Movement Left", "Movement Right"] ("Chnl Names"), 9:w405, 11:w393) -> (15:w414:errorcluster)  [unwired: 1 in, 3 out]
          n236 = case shown="True" w409 {
            tunnel: w408 -> [_ w434]
            tunnel: w407 -> [w425 w433]
            tunnel: w406 -> [w424 w432]
            tunnel: w405 -> [_ w431]
            tunnel: [w425 w428] -> w404
            tunnel: [w424 w427] -> w403
            frame False {
            }
            frame True {
              n237 = Flush Queue(queue=w433, error in (no error)=w432) -> (queue out=w436:refnum<queue>, remaining elements=w429:cluster{"data":waveform(dbl)[]}[], error out=w435:errorcluster)
              n238 = call <vilib>:"Read Self Enqueuer.vi"("Actor"=w434) -> ("Self Enqueuer"=w430:refnum<class "Message Enqueuer.lvclass">)  [unwired: 10 in]
              n239 = Enqueue Element(queue=w436, element=w431, timeout in ms (-1)=0, error in (no error)=w435) -> (queue out=w428:refnum<queue>, error out=w427:errorcluster)  [unwired: 1 out]
              n240 = call "Send Process Live Data Q Mov.vi"("Live Data Q Elements"=w429, "Message Enqueuer in"=w430) -> ()  [unwired: 8 in, 2 out]
            }
          }
          n241 = case shown="Error .." w414 {
            selector: w414 -> [_ w437]
            tunnel: w412 -> [_ w438]
            frame No Error {
            }
            frame Error {
              n242 = Generate User Event(user event=w438, event data cluster=TRUE ("event data")) -> ()  [unwired: 2 in, 2 out]
              n243 = call <vilib>:"Simple Error Handler.vi"("error in (no error)"=w437) -> ()  [unwired: 4 in, 5 out]
            }
          }
        }
        n244 = call <vilib>:"DAQmx Stop Task.vi"("task/channels in"=w363) -> ()  [unwired: 13 in, 2 out]
        n245 = Release Queue(queue=w357, error in (no error)=w355) -> (error out=w358:errorcluster)  [unwired: 1 in, 2 out]
        n246 = Release Queue(queue=w344, error in (no error)=w342) -> (error out=w343:errorcluster)  [unwired: 1 in, 2 out]
        n247 = Enqueue Element(queue=w365, element=waveform(dbl)[] [] ("data"), error in (no error)=w354) -> ()  [unwired: 1 in, 3 out]
        n248 = call <vilib>:"Simple Error Handler.vi"("error in (no error)"=w358) -> ()  [unwired: 4 in, 5 out]
        n249 = call <vilib>:"Simple Error Handler.vi"("error in (no error)"=w343) -> ()  [unwired: 4 in, 5 out]
      }
      frame "Acquire Force and EMG" {
        # "Refresh rate"
        n250 = in-place {
          in-place-border: [w532] -> w502
          in-place-border: [w531] -> w501
          in-place-border: [w528] -> w500
          in-place-border: [w527] -> w499
          in-place-border: [w526] -> w498
          in-place-border: [w525] -> w491
          in-place-border: [w520] -> w480
          n251 = in-place-cluster #13(w503) -> ("Task Ref"=w538:refnum<vi>, "Force Calibration"=w536:refnum<vi>, "TDMS File"=w533:refnum<vi>, "Trial Num"=w530:refnum<vi>, "Shut Down"=w527:refnum<user-event>, "Force Rate Hz"=w524:refnum<vi>, "Decimation factor"=w522:refnum<vi>)
          n252 = property class="DigNum (strict)"(reference=w524) -> (reference out=w523:refnum<vi>, "Value"=w525:u16)  [unwired: 1 in, 1 out]
          n253 = property class="DigNum (strict)"(reference=w522) -> (reference out=w521:refnum<vi>, "Value"=w520:i32)  [unwired: 1 in, 1 out]
          n254 = property class="DAQmxName (strict)"(reference=w538) -> (reference out=w537:refnum<vi>, "Value"=w532:refnum<k21>)  [unwired: 1 in, 1 out]
          n255 = property class="DigNum (strict)"(reference=w530) -> (reference out=w529:refnum<vi>, "Value"=w528:i32)  [unwired: 1 in, 1 out]
          n256 = property class="Clust (strict)"(reference=w536) -> (reference out=w535:refnum<vi>, "Value"=w526:cluster{"Left":dbl, "Right":dbl})  [unwired: 1 in, 1 out]
          n257 = property class="Ref (strict)"(reference=w533) -> (reference out=w534:refnum<vi>, "Value"=w531:refnum<k34>)  [unwired: 1 in, 1 out]
          n258 = in-place-cluster #13("Task Ref"=w537, "Force Calibration"=w535, "TDMS File"=w534, "Trial Num"=w529, "Shut Down"=w527, "Force Rate Hz"=w523, "Decimation factor"=w521) -> (w495:refnum<class "NI Force Task.lvclass">)
        }
        n259 = Divide(x=w491, y=u16 30) -> (x/y=w493:dbl)
        n260 = Round To Nearest(number=w493) -> (nearest integer value=w487:dbl)
        n261 = Obtain Queue(max queue size (-1, unlimited)=w487, name (unnamed)="NI Data Plot Q", element data type=waveform(dbl)[] [] ("data")) -> (queue out=w488:refnum<queue>, error out=w483:errorcluster)  [unwired: 2 in, 1 out]
        n262 = Number To Fractional String(number=w500, precision (6)=i16 0) -> (F-format string=w485:string)  [unwired: 2 in]
        n263 = Obtain Queue(name (unnamed)="Data Q", element data type=waveform(dbl)[] [] ("data")) -> (queue out=w515:refnum<queue>, error out=w506:errorcluster)  [unwired: 3 in, 1 out]
        n264 = Unbundle By Name(w498) -> ("Left"=w497:dbl, "Right"=w496:dbl)
        n265 = Concatenate Strings("EMG Trial " ("string"), w485) -> (w509:string)
        n266 = Divide(x=w480, y=2000.0) -> (x/y=w482:dbl)
        n267 = call <vilib>:"DAQmx Start Task.vi"("task/channels in"=w502) -> ("task out"=w519:refnum<k21>, "error out"=w518:errorcluster)  [unwired: 13 in]
        n268 = Concatenate Strings("Force Trial " ("string"), w485) -> (w484:string)
        n269 = while {
          tunnel: w515 -> [w567]
          tunnel: w509 -> [w565]
          tunnel: [w564] -> w507
          tunnel: w506 -> [w563]
          tunnel: [w562] -> w505
          tunnel: w501 -> [w560]
          tunnel: w499 -> [w559]
          tunnel: w497 -> [w558]
          tunnel: w496 -> [w557]
          tunnel: w495 -> [w547]
          tunnel: [w546] -> w494
          tunnel: w488 -> [w545]
          tunnel: w480 -> [w550]
          tunnel: w484 -> [w549]
          tunnel: w483 -> [w542]
          tunnel: w482 -> [w541]
          stop <- w566 stop-if-true
          n270 = Dequeue Element(queue=w567, error in (no error)=w563) -> (queue out=w564:refnum<queue>, element=w552:waveform(dbl)[], error out=w562:errorcluster)  [unwired: 1 in, 1 out]
          n271 = in-place {
            in-place-border: [w616] -> w571
            in-place-border: w558 -> [w622]
            in-place-border: w557 -> [w624]
            in-place-border: w550 -> [w623]
            in-place-border: [w611] -> w548
            in-place-border: [w613] -> w544
            in-place-border: [w619] -> w543
            in-place-border: [w616] -> w540
            n272 = in-place-split #14(w552, 2) -> (w618:waveform(dbl)[], w613:waveform(dbl)[])
            n273 = in-place {
              in-place-border: w624 -> [w636]
              in-place-border: w623 -> [w631]
              in-place-border: w622 -> [w635]
              in-place-border: [w632] -> w619
              in-place-border: [w630] -> w617
              n274 = in-place-array #15(w618, 0, 1) -> (w634:waveform(dbl), w630:waveform(dbl))
              n275 = in-place-array #16(w613, 2, 3) -> (w628:waveform(dbl), w627:waveform(dbl))
              n276 = in-place {
                in-place-border: w636 -> [w651]
                in-place-border: w631 -> [w637]
                in-place-border: w635 -> [w647]
                in-place-border: [w644] -> w632
                w640 = TRUE ("averaging")
                n277 = in-place-cluster #17(w634) -> ("Y"=w650:dbl[])
                n278 = in-place-cluster #18(w630) -> ("Y"=w648:dbl[])
                n279 = in-place-cluster #19(w628) -> ("Y"=w642:dbl[])
                n280 = in-place-cluster #20(w627) -> ("Y"=w641:dbl[])
                n281 = call-poly <vilib>:"Decimate (continuous).vi"("averaging"=w640, "decimating factor"=w637, "X"=w650) -> ("Decimated Array"=w649:dbl[])  [unwired: 7 in, 1 out]
                n282 = call-poly <vilib>:"Decimate (continuous).vi"("averaging"=w640, "decimating factor"=w637, "X"=w648) -> ("Decimated Array"=w643:dbl[])  [unwired: 7 in, 1 out]
                n283 = call-poly <vilib>:"Decimate (continuous).vi"("averaging"=w640, "decimating factor"=w637, "X"=w642) -> ("Decimated Array"=w639:dbl[])  [unwired: 7 in, 1 out]
                n284 = call-poly <vilib>:"Decimate (continuous).vi"("averaging"=w640, "decimating factor"=w637, "X"=w641) -> ("Decimated Array"=w638:dbl[])  [unwired: 7 in, 1 out]
                n285 = Subtract(x=w649, y=w647) -> (x-y=w646:dbl[])
                n286 = Subtract(x=w643, y=w651) -> (x-y=w645:dbl[])
                n287 = Empty Array?(array=w643) -> (empty?=w644:bool)
                n288 = in-place-cluster #17("Y"=w646) -> (w633:waveform(dbl))
                n289 = in-place-cluster #18("Y"=w645) -> (w629:waveform(dbl))
                n290 = in-place-cluster #19("Y"=w639) -> (w626:waveform(dbl))
                n291 = in-place-cluster #20("Y"=w638) -> (w625:waveform(dbl))
              }
              n292 = in-place-array #15(w633, w629) -> (w611:waveform(dbl)[])  [unwired: 2 out]
              n293 = in-place-array #16(w626, w625) -> (w612:waveform(dbl)[])  [unwired: 2 out]
            }
            n294 = call-poly <vilib>:"Get Waveform Time Array.vi"("waveform in"=w617) -> ("X array"=w616:timestamp[])  [unwired: 9 in, 1 out]
            n295 = in-place-split #14(w611, w612) -> (w539:waveform(dbl)[])  [unwired: 1 out]
          }
          n296 = Empty Array?(array=w552) -> (empty?=w566:bool)
          n297 = TDMS Write(0:w560, 5:w565, 7:string[] ["Time stamp"] ("channel name(s) in (Untitled)"), 9:w571) -> (4:w569:refnum<k34>, 6:w568:string, 15:w561:errorcluster)  [unwired: 2 in, 1 out]
          n298 = TDMS Write(0:w569, 5:w568, 7:string[] ["EMG Left", "EMG Right"] ("Chnl Names"), 9:w544, 11:w561) -> (4:w556:refnum<k34>, 15:w555:errorcluster)  [unwired: 1 in, 2 out]
          n299 = case shown="False" w543 {
            tunnel: w556 -> [w580 _]
            tunnel: w555 -> [w584 w608]
            tunnel: [w594 w608] -> w553
            tunnel: w549 -> [w582 _]
            tunnel: w548 -> [w586 _]
            tunnel: w547 -> [w593 _]
            tunnel: [w592 w607] -> w546
            tunnel: w545 -> [w591 w607]
            tunnel: w542 -> [w585 _]
            tunnel: w541 -> [w575 _]
            tunnel: w540 -> [w577 _]
            tunnel: w539 -> [w572 _]
            frame False {
              n300 = To Double Precision Float(number=w577) -> (double precision float=w576:dbl[])
              n301 = Subtract(x=w576, y=w575) -> (x-y=w574:dbl[])
              n302 = Enqueue Element(queue=w591, element=w572, timeout in ms (-1)=0, error in (no error)=w585) -> (queue out=w590:refnum<queue>, timed out?=w589:bool, error out=w588:errorcluster)
              n303 = To Time Stamp(1:w574) -> (0:w573:timestamp[])
              n304 = case shown="True" w589 {
                tunnel: w593 -> [_ w604]
                tunnel: w590 -> [w596 w603]
                tunnel: w588 -> [_ w602]
                tunnel: [w596 w599] -> w592
                tunnel: w572 -> [_ w597]
                frame False {
                }
                frame True {
                  n305 = Flush Queue(queue=w603, error in (no error)=w602) -> (queue out=w606:refnum<queue>, remaining elements=w600:cluster{"data":waveform(dbl)[]}[], error out=w605:errorcluster)
                  n306 = call <vilib>:"Read Self Enqueuer.vi"("Actor"=w604) -> ("Self Enqueuer"=w601:refnum<class "Message Enqueuer.lvclass">)  [unwired: 10 in]
                  n307 = Enqueue Element(queue=w606, element=w597, timeout in ms (-1)=0, error in (no error)=w605) -> (queue out=w599:refnum<queue>)  [unwired: 2 out]
                  n308 = call "Send Process Live Data Q.vi"("Live Data Q Elements"=w600, "Message Enqueuer in"=w601) -> ()  [unwired: 8 in, 2 out]
                }
              }
              n309 = TDMS Write(0:w580, 5:w582, 7:string[] ["Time"] ("channel name(s) in (Untitled)"), 9:w573, 11:w584) -> (4:w579:refnum<k34>, 6:w581:string, 15:w583:errorcluster)  [unwired: 1 in, 1 out]
              n310 = TDMS Write(0:w579, 5:w581, 7:string[] ["Raw Force Left", "Raw Force Right"] ("Chnl Names"), 9:w586, 11:w583) -> (15:w594:errorcluster)  [unwired: 1 in, 3 out]
            }
            frame True {
            }
          }
          n311 = case shown="Error .." w553 {
            tunnel: w559 -> [_ w609]
            frame No Error {
            }
            frame Error {
              n312 = Generate User Event(user event=w609, event data cluster=TRUE ("event data")) -> ()  [unwired: 2 in, 2 out]
            }
          }
        }
        n313 = while {
          tunnel: w519 -> [w663]
          tunnel: w518 -> [w662]
          tunnel: w515 -> [w660]
          tunnel: [w659] -> w512
          tunnel: [w657] -> w514
          tunnel: [w654] -> w504
          tunnel: w499 -> [w653]
          stop <- w656 stop-if-true
          n314 = call-poly <vilib>:"DAQmx Read.vi"("task/channels in"=w663, "error in"=w662) -> ("task out"=w659:refnum<k21>, "data"=w658:waveform(dbl)[], "error out"=w661:errorcluster)  [unwired: 11 in]
          n315 = case shown="No Error" w661 {
            selector: w661 -> [_ w671]
            tunnel: w660 -> [w668 w674]
            tunnel: w658 -> [w667 _]
            tunnel: [w666 w674] -> w657
            tunnel: [FALSE ("x") w672] -> w655
            tunnel: [w664 errorcluster {"status"=FALSE, "code"=0, "source"=""} ("error out")] -> w654
            tunnel: w653 -> [_ w669]
            frame No Error {
              n316 = Enqueue Element(queue=w668, element=w667) -> (queue out=w666:refnum<queue>, error out=w664:errorcluster)  [unwired: 2 in, 1 out]
            }
            frame Error {
              n317 = Generate User Event(user event=w669, event data cluster=TRUE ("event data")) -> ()  [unwired: 2 in, 2 out]
              n318 = Unbundle By Name(w671) -> ("status"=w672:bool)
            }
          }
          n319 = local read "Stop Acquire"() -> (w652:bool)
          n320 = Or(x=w655, y=w652) -> (x .or. y?=w656:bool)
        }
        n321 = call <vilib>:"DAQmx Stop Task.vi"("task/channels in"=w512) -> ()  [unwired: 13 in, 2 out]
        n322 = Enqueue Element(queue=w514, element=waveform(dbl)[] [] ("data"), error in (no error)=w504) -> ()  [unwired: 1 in, 3 out]
        n323 = Release Queue(queue=w507, error in (no error)=w505) -> (error out=w508:errorcluster)  [unwired: 1 in, 2 out]
        n324 = Release Queue(queue=w494) -> ()  [unwired: 2 in, 3 out]
        n325 = call <vilib>:"Simple Error Handler.vi"("error in (no error)"=w508) -> ()  [unwired: 4 in, 5 out]
      }
      frame "Acquire Movement and EMG" {
        # "Refresh rate"
        n326 = in-place {
          in-place-border: [w732] -> w699
          in-place-border: [w731] -> w698
          in-place-border: [w728] -> w697
          in-place-border: [w727] -> w696
          in-place-border: [w726] -> w695
          in-place-border: [w725] -> w688
          in-place-border: [w720] -> w677
          in-place-border: [w717] -> w676
          n327 = in-place-cluster #21(w700) -> ("Task Ref"=w738:refnum<vi>, "Force Calibration"=w736:refnum<vi>, "TDMS File"=w733:refnum<vi>, "Trial Num"=w730:refnum<vi>, "Shut Down"=w727:refnum<user-event>, "Force Rate Hz"=w724:refnum<vi>, "Decimation factor"=w722:refnum<vi>, "Task Info In"=w719:refnum<vi>)
          n328 = property class="DigNum (strict)"(reference=w724) -> (reference out=w723:refnum<vi>, "Value"=w725:u16)  [unwired: 1 in, 1 out]
          n329 = property class="DigNum (strict)"(reference=w722) -> (reference out=w721:refnum<vi>, "Value"=w720:i32)  [unwired: 1 in, 1 out]
          n330 = property class="DAQmxName (strict)"(reference=w738) -> (reference out=w737:refnum<vi>, "Value"=w732:refnum<k21>)  [unwired: 1 in, 1 out]
          n331 = property class="DigNum (strict)"(reference=w730) -> (reference out=w729:refnum<vi>, "Value"=w728:i32)  [unwired: 1 in, 1 out]
          n332 = property class="Clust (strict)"(reference=w736) -> (reference out=w735:refnum<vi>, "Value"=w726:cluster{"Left":dbl, "Right":dbl})  [unwired: 1 in, 1 out]
          n333 = property class="Ref (strict)"(reference=w733) -> (reference out=w734:refnum<vi>, "Value"=w731:refnum<k34>)  [unwired: 1 in, 1 out]
          n334 = property class="Clust (strict)"(reference=w719) -> (reference out=w718:refnum<vi>, "Value"=w717:T1)  [unwired: 1 in, 1 out]
          n335 = in-place-cluster #21("Task Ref"=w737, "Force Calibration"=w735, "TDMS File"=w734, "Trial Num"=w729, "Shut Down"=w727, "Force Rate Hz"=w723, "Decimation factor"=w721, "Task Info In"=w718) -> (w692:refnum<class "NI Force Task.lvclass">)
        }
        n336 = Divide(x=w688, y=u16 30) -> (x/y=w690:dbl)
        n337 = Round To Nearest(number=w690) -> (nearest integer value=w684:dbl)
        n338 = Obtain Queue(max queue size (-1, unlimited)=w684, name (unnamed)="NI Data Plot Q", element data type=waveform(dbl)[] [] ("data")) -> (queue out=w685:refnum<queue>, error out=w680:errorcluster)  [unwired: 2 in, 1 out]
        n339 = Number To Fractional String(number=w697, precision (6)=i16 0) -> (F-format string=w682:string)  [unwired: 2 in]
        n340 = Unbundle By Name(w676) -> ("Adjusted MVC (N)"=w675:dbl)
        n341 = Obtain Queue(name (unnamed)="Data Q", element data type=waveform(dbl)[] [] ("data")) -> (queue out=w712:refnum<queue>, error out=w703:errorcluster)  [unwired: 3 in, 1 out]
        n342 = Unbundle By Name(w695) -> ("Left"=w694:dbl, "Right"=w693:dbl)
        n343 = Concatenate Strings("EMG Trial " ("string"), w682) -> (w706:string)
        n344 = Divide(x=w677, y=2000.0) -> (x/y=w679:dbl)
        n345 = call <vilib>:"DAQmx Start Task.vi"("task/channels in"=w699) -> ("task out"=w716:refnum<k21>, "error out"=w715:errorcluster)  [unwired: 13 in]
        n346 = Concatenate Strings("Movement Trial " ("string"), w682) -> (w681:string)
        n347 = while {
          tunnel: w712 -> [w770]
          tunnel: w706 -> [w768]
          tunnel: [w767] -> w704
          tunnel: w703 -> [w766]
          tunnel: [w765] -> w702
          tunnel: w698 -> [w763]
          tunnel: w696 -> [w762]
          tunnel: w694 -> [w761]
          tunnel: w693 -> [w760]
          tunnel: w692 -> [w750]
          tunnel: [w749] -> w691
          tunnel: w685 -> [w748]
          tunnel: w677 -> [w753]
          tunnel: w681 -> [w752]
          tunnel: w680 -> [w745]
          tunnel: w679 -> [w744]
          tunnel: w675 -> [w741]
          stop <- w769 stop-if-true
          n348 = Dequeue Element(queue=w770, error in (no error)=w766) -> (queue out=w767:refnum<queue>, element=w755:waveform(dbl)[], error out=w765:errorcluster)  [unwired: 1 in, 1 out]
          n349 = in-place {
            in-place-border: [w830] -> w774
            in-place-border: w761 -> [w835]
            in-place-border: w760 -> [w837]
            in-place-border: w753 -> [w836]
            in-place-border: [w825] -> w751
            in-place-border: [w827] -> w747
            in-place-border: [w832] -> w746
            in-place-border: [w830] -> w743
            in-place-border: w741 -> [w824]
            in-place-border: [w822] -> w740
            in-place-border: [w821] -> w739
            n350 = in-place-split #22(w755, 2) -> (w823:waveform(dbl)[], w827:waveform(dbl)[])
            n351 = in-place {
              in-place-border: w837 -> [w852]
              in-place-border: w836 -> [w848]
              in-place-border: w835 -> [w851]
              in-place-border: [w849] -> w832
              in-place-border: [w840] -> w831
              in-place-border: w824 -> [w842]
              in-place-border: [w839] -> w822
              in-place-border: [w838] -> w821
              n352 = in-place-array #23(w823, 0, 1) -> (w841:waveform(dbl), w840:waveform(dbl))
              n353 = in-place-array #24(w827, 2, 3) -> (w846:waveform(dbl), w845:waveform(dbl))
              n354 = in-place {
                in-place-border: w852 -> [w870]
                in-place-border: w848 -> [w860]
                in-place-border: w851 -> [w867]
                in-place-border: [w866] -> w849
                in-place-border: w842 -> [w855]
                w863 = TRUE ("averaging")
                n355 = in-place-cluster #25(w841) -> ()  [unwired: 1 out]
                n356 = in-place-cluster #26(w840) -> ()  [unwired: 1 out]
                n357 = in-place-cluster #27(w841) -> ("Y"=w869:dbl[])
                n358 = in-place-cluster #28(w840) -> ("Y"=w868:dbl[])
                n359 = in-place-cluster #29(w846) -> ("Y"=w865:dbl[])
                n360 = in-place-cluster #30(w845) -> ("Y"=w864:dbl[])
                n361 = call-poly <vilib>:"Decimate (continuous).vi"("averaging"=w863, "decimating factor"=w860, "X"=w869) -> ("Decimated Array"=w854:dbl[])  [unwired: 7 in, 1 out]
                n362 = call-poly <vilib>:"Decimate (continuous).vi"("averaging"=w863, "decimating factor"=w860, "X"=w868) -> ("Decimated Array"=w853:dbl[])  [unwired: 7 in, 1 out]
                n363 = call-poly <vilib>:"Decimate (continuous).vi"("averaging"=w863, "decimating factor"=w860, "X"=w865) -> ("Decimated Array"=w862:dbl[])  [unwired: 7 in, 1 out]
                n364 = call-poly <vilib>:"Decimate (continuous).vi"("averaging"=w863, "decimating factor"=w860, "X"=w864) -> ("Decimated Array"=w861:dbl[])  [unwired: 7 in, 1 out]
                n365 = Subtract(x=w854, y=w867) -> (x-y=w859:dbl[])
                n366 = Subtract(x=w853, y=w870) -> (x-y=w858:dbl[])
                n367 = Multiply(x=w859, y=w855) -> (x*y=w856:dbl[])
                n368 = Empty Array?(array=w853) -> (empty?=w866:bool)
                n369 = Multiply(x=w855, y=w858) -> (x*y=w857:dbl[])
                n370 = in-place-cluster #25("Y"=w854) -> (w839:waveform(dbl))
                n371 = in-place-cluster #26("Y"=w853) -> (w838:waveform(dbl))
                n372 = in-place-cluster #27("Y"=w856) -> (w850:waveform(dbl))
                n373 = in-place-cluster #28("Y"=w857) -> (w847:waveform(dbl))
                n374 = in-place-cluster #29("Y"=w862) -> (w844:waveform(dbl))
                n375 = in-place-cluster #30("Y"=w861) -> (w843:waveform(dbl))
              }
              n376 = in-place-array #23(w850, w847) -> (w825:waveform(dbl)[])  [unwired: 2 out]
              n377 = in-place-array #24(w844, w843) -> (w826:waveform(dbl)[])  [unwired: 2 out]
            }
            n378 = call-poly <vilib>:"Get Waveform Time Array.vi"("waveform in"=w831) -> ("X array"=w830:timestamp[])  [unwired: 9 in, 1 out]
            n379 = in-place-split #22(w825, w826) -> (w742:waveform(dbl)[])  [unwired: 1 out]
          }
          n380 = Empty Array?(array=w755) -> (empty?=w769:bool)
          n381 = TDMS Write(0:w763, 5:w768, 7:string[] ["Time stamp"] ("channel name(s) in (Untitled)"), 9:w774) -> (4:w772:refnum<k34>, 6:w771:string, 15:w764:errorcluster)  [unwired: 2 in, 1 out]
          n382 = TDMS Write(0:w772, 5:w771, 7:string[] ["EMG Left", "EMG Right"] ("Chnl Names"), 9:w747, 11:w764) -> (4:w759:refnum<k34>, 15:w758:errorcluster)  [unwired: 1 in, 2 out]
          n383 = case shown="False" w746 {
            tunnel: w759 -> [w792 _]
            tunnel: w758 -> [w796 w818]
            tunnel: [w780 w818] -> w756
            tunnel: w752 -> [w794 _]
            tunnel: w751 -> [w778 _]
            tunnel: w750 -> [w804 _]
            tunnel: [w803 w817] -> w749
            tunnel: w748 -> [w802 w817]
            tunnel: w745 -> [w797 _]
            tunnel: w744 -> [w787 _]
            tunnel: w743 -> [w789 _]
            tunnel: w742 -> [w784 _]
            tunnel: w740 -> [w777 _]
            tunnel: w739 -> [w776 _]
            frame False {
              n384 = To Double Precision Float(number=w789) -> (double precision float=w788:dbl[])
              n385 = Subtract(x=w788, y=w787) -> (x-y=w786:dbl[])
              n386 = Enqueue Element(queue=w802, element=w784, timeout in ms (-1)=0, error in (no error)=w797) -> (queue out=w801:refnum<queue>, timed out?=w800:bool, error out=w799:errorcluster)
              n387 = Build Array(w777, w776) -> (w775:waveform(dbl)[])
              n388 = To Time Stamp(1:w786) -> (0:w785:timestamp[])
              n389 = case shown="True" w800 {
                tunnel: w804 -> [_ w814]
                tunnel: w801 -> [w806 w813]
                tunnel: w799 -> [_ w812]
                tunnel: [w806 w809] -> w803
                tunnel: w784 -> [_ w807]
                frame False {
                }
                frame True {
                  n390 = Flush Queue(queue=w813, error in (no error)=w812) -> (queue out=w816:refnum<queue>, remaining elements=w810:cluster{"data":waveform(dbl)[]}[], error out=w815:errorcluster)
                  n391 = call <vilib>:"Read Self Enqueuer.vi"("Actor"=w814) -> ("Self Enqueuer"=w811:refnum<class "Message Enqueuer.lvclass">)  [unwired: 10 in]
                  n392 = Enqueue Element(queue=w816, element=w807, timeout in ms (-1)=0, error in (no error)=w815) -> (queue out=w809:refnum<queue>)  [unwired: 2 out]
                  n393 = call "Send Process Live Data Q Mov.vi"("Live Data Q Elements"=w810, "Message Enqueuer in"=w811) -> ()  [unwired: 8 in, 2 out]
                }
              }
              n394 = TDMS Write(0:w792, 5:w794, 7:string[] ["Time"] ("channel name(s) in (Untitled)"), 9:w785, 11:w796) -> (4:w791:refnum<k34>, 6:w793:string, 15:w795:errorcluster)  [unwired: 1 in, 1 out]
              n395 = TDMS Write(0:w791, 5:w793, 7:string[] ["Raw Potentiometer Left", "Raw Potentiometer Right"] ("Chnl Names"), 9:w775, 11:w795) -> (4:w781:refnum<k34>, 6:w782:string, 15:w779:errorcluster)  [unwired: 1 in, 1 out]
              n396 = TDMS Write(0:w781, 5:w782, 7:string[] ["Potentiometer Left", "Potentiometer Right"] ("Chnl Names"), 9:w778, 11:w779) -> (15:w780:errorcluster)  [unwired: 1 in, 3 out]
            }
            frame True {
            }
          }
          n397 = case shown="No Error" w756 {
            tunnel: w762 -> [_ w819]
            frame No Error {
            }
            frame Error {
              n398 = Generate User Event(user event=w819, event data cluster=TRUE ("event data")) -> ()  [unwired: 2 in, 2 out]
            }
          }
        }
        n399 = while {
          tunnel: w716 -> [w882]
          tunnel: w715 -> [w881]
          tunnel: w712 -> [w879]
          tunnel: [w878] -> w709
          tunnel: [w876] -> w711
          tunnel: [w873] -> w701
          tunnel: w696 -> [w872]
          stop <- w875 stop-if-true
          n400 = call-poly <vilib>:"DAQmx Read.vi"("task/channels in"=w882, "error in"=w881) -> ("task out"=w878:refnum<k21>, "data"=w877:waveform(dbl)[], "error out"=w880:errorcluster)  [unwired: 11 in]
          n401 = case shown="No Error" w880 {
            selector: w880 -> [_ w890]
            tunnel: w879 -> [w887 w893]
            tunnel: w877 -> [w886 _]
            tunnel: [w885 w893] -> w876
            tunnel: [FALSE ("x") w891] -> w874
            tunnel: [w883 errorcluster {"status"=FALSE, "code"=0, "source"=""} ("error out")] -> w873
            tunnel: w872 -> [_ w888]
            frame No Error {
              n402 = Enqueue Element(queue=w887, element=w886) -> (queue out=w885:refnum<queue>, error out=w883:errorcluster)  [unwired: 2 in, 1 out]
            }
            frame Error {
              n403 = Generate User Event(user event=w888, event data cluster=TRUE ("event data")) -> ()  [unwired: 2 in, 2 out]
              n404 = Unbundle By Name(w890) -> ("status"=w891:bool)
            }
          }
          n405 = local read "Stop Acquire"() -> (w871:bool)
          n406 = Or(x=w874, y=w871) -> (x .or. y?=w875:bool)
        }
        n407 = call <vilib>:"DAQmx Stop Task.vi"("task/channels in"=w709) -> ()  [unwired: 13 in, 2 out]
        n408 = Enqueue Element(queue=w711, element=waveform(dbl)[] [] ("data"), error in (no error)=w701) -> ()  [unwired: 1 in, 3 out]
        n409 = Release Queue(queue=w704, error in (no error)=w702) -> (error out=w705:errorcluster)  [unwired: 1 in, 2 out]
        n410 = Release Queue(queue=w691) -> ()  [unwired: 2 in, 3 out]
        n411 = call <vilib>:"Simple Error Handler.vi"("error in (no error)"=w705) -> ()  [unwired: 4 in, 5 out]
      }
      frame "Collect EMG only" {
        n412 = in-place {
          in-place-border: [w930] -> w907
          in-place-border: [w929] -> w906
          in-place-border: [w926] -> w905
          in-place-border: [w925] -> w904
          n413 = in-place-cluster #31(w908) -> ("Task Ref"=w934:refnum<vi>, "TDMS File"=w931:refnum<vi>, "Trial Num"=w928:refnum<vi>, "Shut Down"=w925:refnum<user-event>)
          n414 = property class="DAQmxName (strict)"(reference=w934) -> (reference out=w933:refnum<vi>, "Value"=w930:refnum<k21>)  [unwired: 1 in, 1 out]
          n415 = property class="DigNum (strict)"(reference=w928) -> (reference out=w927:refnum<vi>, "Value"=w926:i32)  [unwired: 1 in, 1 out]
          n416 = property class="Ref (strict)"(reference=w931) -> (reference out=w932:refnum<vi>, "Value"=w929:refnum<k34>)  [unwired: 1 in, 1 out]
          n417 = in-place-cluster #31("Task Ref"=w933, "TDMS File"=w932, "Trial Num"=w927, "Shut Down"=w925) -> (w903:refnum<class "NI Force Task.lvclass">)
        }
        n418 = Number To Fractional String(number=w905, precision (6)=i16 0) -> (F-format string=w902:string)  [unwired: 2 in]
        n419 = Obtain Queue(name (unnamed)="Data Q", element data type=waveform(dbl)[] [] ("data")) -> (queue out=w920:refnum<queue>, error out=w911:errorcluster)  [unwired: 3 in, 1 out]
        n420 = Obtain Queue(max queue size (-1, unlimited)=35, name (unnamed)="NI Data Plot Q", element data type=waveform(dbl)[] [] ("data")) -> (queue out=w898:refnum<queue>, error out=w897:errorcluster)  [unwired: 2 in, 1 out]
        n421 = Concatenate Strings("Parabola Num " ("string"), w902) -> (w914:string)
        n422 = call <vilib>:"DAQmx Start Task.vi"("task/channels in"=w907) -> ("task out"=w924:refnum<k21>, "error out"=w923:errorcluster)  [unwired: 13 in]
        n423 = while {
          tunnel: w920 -> [w957]
          tunnel: w914 -> [w955]
          tunnel: [w954] -> w912
          tunnel: w911 -> [w953]
          tunnel: [w952] -> w910
          tunnel: w906 -> [w950]
          tunnel: w904 -> [w949]
          tunnel: w903 -> [w937]
          tunnel: w898 -> [w940]
          tunnel: w897 -> [w939]
          tunnel: [w936] -> w895
          tunnel: [w935] -> w894
          stop <- w956 stop-if-true
          n424 = Dequeue Element(queue=w957, error in (no error)=w953) -> (queue out=w954:refnum<queue>, element=w947:waveform(dbl)[], error out=w952:errorcluster)  [unwired: 1 in, 1 out]
          n425 = in-place {
            in-place-border: [w978] -> w961
            n426 = in-place-array #32(w947, 0) -> (w977:waveform(dbl))
            n427 = call-poly <vilib>:"Get Waveform Time Array.vi"("waveform in"=w977) -> ("X array"=w978:timestamp[])  [unwired: 9 in, 1 out]
            n428 = in-place-array #32(w977) -> (w938:waveform(dbl)[])  [unwired: 1 out]
          }
          n429 = Empty Array?(array=w947) -> (empty?=w956:bool)
          n430 = TDMS Write(0:w950, 5:w955, 7:string[] ["Time stamp"] ("channel name(s) in (Untitled)"), 9:w961) -> (4:w959:refnum<k34>, 6:w958:string, 15:w951:errorcluster)  [unwired: 2 in, 1 out]
          n431 = Enqueue Element(queue=w940, element=w938, timeout in ms (-1)=0, error in (no error)=w939) -> (queue out=w943:refnum<queue>, timed out?=w944:bool, error out=w942:errorcluster)
          n432 = TDMS Write(0:w959, 5:w958, 7:string[] ["S1 Left", "S1 Right", "S2 Left", "S2 Right", "S3 Left", "S3 Right", "S4 Left", "S4 Right", "S5 Left", "S5 Right", "S6 Left", "S6 Right", "S7 Left", "S7 Right", "S8 Left", "S8 Right"] ("Chnl Names"), 9:w938, 11:w951) -> (15:w945:errorcluster)  [unwired: 1 in, 3 out]
          n433 = case shown="True" w944 {
            tunnel: w937 -> [_ w972]
            tunnel: w943 -> [w963 w971]
            tunnel: w942 -> [w962 w970]
            tunnel: w938 -> [_ w969]
            tunnel: [w963 w968] -> w936
            tunnel: [w962 w967] -> w935
            frame False {
            }
            frame True {
              n434 = Flush Queue(queue=w971, error in (no error)=w970) -> (queue out=w974:refnum<queue>, remaining elements=w965:cluster{"data":waveform(dbl)[]}[], error out=w973:errorcluster)
              n435 = call <vilib>:"Read Self Enqueuer.vi"("Actor"=w972) -> ("Self Enqueuer"=w964:refnum<class "Message Enqueuer.lvclass">)  [unwired: 10 in]
              n436 = Enqueue Element(queue=w974, element=w969, timeout in ms (-1)=0, error in (no error)=w973) -> (queue out=w968:refnum<queue>, error out=w967:errorcluster)  [unwired: 1 out]
              n437 = call "Send Process Live Data Q EMG.vi"("Live Data Q Elements"=w965, "Message Enqueuer in"=w964) -> ()  [unwired: 8 in, 2 out]
            }
          }
          n438 = case shown="Error .." w945 {
            tunnel: w949 -> [_ w975]
            frame No Error {
            }
            frame Error {
              n439 = Generate User Event(user event=w975, event data cluster=TRUE ("event data")) -> ()  [unwired: 2 in, 2 out]
            }
          }
        }
        n440 = while {
          tunnel: w924 -> [w990]
          tunnel: w923 -> [w989]
          tunnel: w920 -> [w987]
          tunnel: [w986] -> w917
          tunnel: [w984] -> w919
          tunnel: [w981] -> w909
          tunnel: w904 -> [w980]
          stop <- w983 stop-if-true
          n441 = call-poly <vilib>:"DAQmx Read.vi"("task/channels in"=w990, "error in"=w989) -> ("task out"=w986:refnum<k21>, "data"=w985:waveform(dbl)[], "error out"=w988:errorcluster)  [unwired: 11 in]
          n442 = case shown="No Error" w988 {
            selector: w988 -> [_ w998]
            tunnel: w987 -> [w995 w1001]
            tunnel: w985 -> [w994 _]
            tunnel: [w993 w1001] -> w984
            tunnel: [FALSE ("x") w999] -> w982
            tunnel: [w991 errorcluster {"status"=FALSE, "code"=0, "source"=""} ("error out")] -> w981
            tunnel: w980 -> [_ w996]
            frame No Error {
              n443 = Enqueue Element(queue=w995, element=w994) -> (queue out=w993:refnum<queue>, error out=w991:errorcluster)  [unwired: 2 in, 1 out]
            }
            frame Error {
              n444 = Generate User Event(user event=w996, event data cluster=TRUE ("event data")) -> ()  [unwired: 2 in, 2 out]
              n445 = Unbundle By Name(w998) -> ("status"=w999:bool)
            }
          }
          n446 = local read "Stop Acquire"() -> (w979:bool)
          n447 = Or(x=w982, y=w979) -> (x .or. y?=w983:bool)
        }
        n448 = call <vilib>:"DAQmx Stop Task.vi"("task/channels in"=w917) -> ()  [unwired: 13 in, 2 out]
        n449 = Release Queue(queue=w895, error in (no error)=w894) -> (error out=w896:errorcluster)  [unwired: 1 in, 2 out]
        n450 = Enqueue Element(queue=w919, element=waveform(dbl)[] [] ("data"), error in (no error)=w909) -> ()  [unwired: 1 in, 3 out]
        n451 = Release Queue(queue=w912, error in (no error)=w910) -> (error out=w913:errorcluster)  [unwired: 1 in, 2 out]
        n452 = call <vilib>:"Simple Error Handler.vi"("error in (no error)"=w896) -> ()  [unwired: 4 in, 5 out]
        n453 = call <vilib>:"Simple Error Handler.vi"("error in (no error)"=w913) -> ()  [unwired: 4 in, 5 out]
      }
      frame "Collect MVC" {
        n454 = in-place {
          in-place-border: [w1113] -> w1041
          in-place-border: [w1112] -> w1013
          in-place-border: [w1111] -> w1021
          in-place-border: [w1108] -> w1018
          in-place-border: [w1105] -> w1012
          n455 = in-place-cluster #33(w1027) -> ("Force Calibration"=w1107:refnum<vi>, "Task Ref"=w1115:refnum<vi>, "Shut Down"=w1112:refnum<user-event>, "Collect MVC"=w1111:refnum<user-event>, "TDMS File"=w1110:refnum<vi>)
          n456 = property class="Ref (strict)"(reference=w1110) -> (reference out=w1109:refnum<vi>, "Value"=w1108:refnum<k34>)  [unwired: 1 in, 1 out]
          n457 = property class="DAQmxName (strict)"(reference=w1115) -> (reference out=w1114:refnum<vi>, "Value"=w1113:refnum<k21>)  [unwired: 1 in, 1 out]
          n458 = property class="Clust (strict)"(reference=w1107) -> (reference out=w1106:refnum<vi>, "Value"=w1105:cluster{"Left":dbl, "Right":dbl})  [unwired: 1 in, 1 out]
          n459 = in-place-cluster #33("Force Calibration"=w1106, "Task Ref"=w1114, "Shut Down"=w1112, "Collect MVC"=w1111, "TDMS File"=w1109) -> (w1028:refnum<class "NI Force Task.lvclass">)
        }
        n460 = Obtain Queue(name (unnamed)="MVC Q", element data type=waveform(dbl)[] [] ("data")) -> (queue out=w1036:refnum<queue>, error out=w1031:errorcluster)  [unwired: 3 in, 1 out]
        n461 = call <vilib>:"DAQmx Start Task.vi"("task/channels in"=w1041) -> ("task out"=w1040:refnum<k21>, "error out"=w1039:errorcluster)  [unwired: 13 in]
        n462 = while {
          tunnel: w1036 -> [w1063]
          tunnel: w1031 -> [w1062]
          tunnel: [w1060] -> w1030
          tunnel: [w1059] -> w1029
          tunnel: [w1058] -> w1024 mode=concatenating
          tunnel: [w1057] -> w1023 mode=concatenating
          tunnel: w1018 -> [w1053]
          tunnel: "MVC EMG" ("group name in (Untitled)") -> [w1047]
          tunnel: [w1044] -> w1016
          stop <- w1061 stop-if-true
          n463 = Dequeue Element(queue=w1063, error in (no error)=w1062) -> (queue out=w1060:refnum<queue>, element=w1056:waveform(dbl)[], error out=w1059:errorcluster)  [unwired: 1 in, 1 out]
          n464 = Empty Array?(array=w1056) -> (empty?=w1061:bool)
          n465 = in-place {
            in-place-border: [w1069] -> w1058
            in-place-border: [w1068] -> w1057
            in-place-border: [w1065] -> w1054
            in-place-border: [w1064] -> w1048
            n466 = in-place-split #34(w1056, 2) -> (w1067:waveform(dbl)[], w1064:waveform(dbl)[])
            n467 = in-place {
              in-place-border: [w1074] -> w1069
              in-place-border: [w1073] -> w1068
              in-place-border: [w1072] -> w1065
              n468 = in-place-array #35(w1067, 0, 1) -> (w1077:waveform(dbl), w1072:waveform(dbl))
              n469 = in-place {
                in-place-border: [w1079] -> w1074
                in-place-border: [w1078] -> w1073
                n470 = in-place-cluster #36(w1077) -> ("Y"=w1079:dbl[])
                n471 = in-place-cluster #37(w1072) -> ("Y"=w1078:dbl[])
                n472 = in-place-cluster #36("Y"=w1079) -> (w1076:waveform(dbl))
                n473 = in-place-cluster #37("Y"=w1078) -> (w1075:waveform(dbl))
              }
              n474 = in-place-array #35(w1076, w1075) -> (w1066:waveform(dbl)[])  [unwired: 2 out]
            }
            n475 = in-place-split #34(w1066, w1064) -> ()  [unwired: 2 out]
          }
          n476 = call-poly <vilib>:"Get Waveform Time Array.vi"("waveform in"=w1054) -> ("X array"=w1051:timestamp[])  [unwired: 9 in, 1 out]
          n477 = TDMS Write(0:w1053, 5:w1047, 7:string[] ["Time Stamp"] ("channel name(s) in (Untitled)"), 9:w1051) -> (4:w1050:refnum<k34>, 6:w1049:string, 15:w1046:errorcluster)  [unwired: 2 in, 1 out]
          n478 = TDMS Write(0:w1050, 5:w1049, 7:string[] ["EMG Left", "EMG Right"] ("Chnl Names"), 9:w1048, 11:w1046) -> (15:w1044:errorcluster)  [unwired: 1 in, 3 out]
        }
        n479 = while {
          tunnel: w1040 -> [w1092]
          tunnel: w1039 -> [w1091]
          tunnel: w1036 -> [w1090]
          tunnel: w1013 -> [w1087]
          tunnel: [w1086] -> w1035
          tunnel: [w1082] -> w1034
          tunnel: [w1081] -> w1033
          tunnel: [w1080] -> w1019
          stop <- w1085 stop-if-true
          n480 = call-poly <vilib>:"DAQmx Read.vi"("task/channels in"=w1092, "error in"=w1091) -> ("task out"=w1086:refnum<k21>, "data"=w1088:waveform(dbl)[], "error out"=w1089:errorcluster)  [unwired: 11 in]
          n481 = case shown="No Error" w1089 {
            selector: w1089 -> [_ w1099]
            tunnel: w1090 -> [w1098 w1104]
            tunnel: w1088 -> [w1097 _]
            tunnel: [w1096 w1104] -> w1082
            tunnel: [FALSE ("x") w1103] -> w1083
            tunnel: w1087 -> [_ w1101]
            tunnel: [w1094 errorcluster {"status"=FALSE, "code"=0, "source"=""} ("error out")] -> w1081
            tunnel: [errorcluster {"status"=FALSE, "code"=0, "source"=""} ("error IO") w1099] -> w1080
            frame No Error {
              n482 = Enqueue Element(queue=w1098, element=w1097) -> (queue out=w1096:refnum<queue>, error out=w1094:errorcluster)  [unwired: 2 in, 1 out]
            }
            frame Error {
              n483 = Generate User Event(user event=w1101, event data cluster=TRUE ("event data")) -> ()  [unwired: 2 in, 2 out]
              n484 = Unbundle By Name(w1099) -> ("status"=w1103:bool)
            }
          }
          n485 = property on="Stop Acquire" class="Bool (strict)"() -> ("Value"=w1084:bool)  [unwired: 2 in, 2 out]
          n486 = Or(x=w1083, y=w1084) -> (x .or. y?=w1085:bool)
        }
        n487 = Unbundle By Name(w1012) -> ("Left"=w1010:dbl, "Right"=w1011:dbl)
        n488 = call <vilib>:"Simple Error Handler.vi"("error in (no error)"=w1019) -> ()  [unwired: 4 in, 5 out]
        n489 = Enqueue Element(queue=w1034, element=waveform(dbl)[] [] ("data"), error in (no error)=w1033) -> ()  [unwired: 1 in, 3 out]
        n490 = expression code="144.74236*x-0.090477"(w1010) -> (w1008:dbl)
        n491 = expression code="142.71878*x-0.08981"(w1011) -> (w1009:dbl)
        n492 = call <vilib>:"DAQmx Stop Task.vi"("task/channels in"=w1035) -> ()  [unwired: 13 in, 2 out]
        n493 = Release Queue(queue=w1030, error in (no error)=w1029) -> ()  [unwired: 1 in, 3 out]
        n494 = Array Max & Min(array=w1024) -> (max value=w1005:dbl)  [unwired: 3 out]
        n495 = Array Max & Min(array=w1023) -> (max value=w1003:dbl)  [unwired: 3 out]
        n496 = expression code="144.74236*x-0.090477"(w1005) -> (w1004:dbl)
        n497 = expression code="142.71878*x-0.08981"(w1003) -> (w1002:dbl)
        n498 = call <vilib>:"Read Caller Enqueuer.vi"("Actor"=w1028) -> ("Caller Enqueuer"=w1026:refnum<class "Message Enqueuer.lvclass">)  [unwired: 10 in]
        n499 = Subtract(x=w1004, y=w1008) -> (x-y=w1007:dbl)
        n500 = Subtract(x=w1002, y=w1009) -> (x-y=w1006:dbl)
        n501 = Bundle(w1007, w1006) -> (w1025:cluster{dbl, dbl})  [unwired: 1 in]
        n502 = call "Send MVC Collection Finished.vi"("Cluster"=w1025, "Message Enqueuer"=w1026) -> ("error out"=w1022:errorcluster)  [unwired: 8 in, 1 out]
        n503 = Generate User Event(user event=w1021, event data cluster=FALSE ("event data"), error in=w1022) -> (error out=w1015:errorcluster)  [unwired: 1 in, 1 out]
        n504 = Merge Errors(w1015, w1016) -> (w1014:errorcluster)
        n505 = case shown="No Error" w1014 {
          tunnel: w1013 -> [_ w1043]
          frame No Error {
          }
          frame Error {
            n506 = Generate User Event(user event=w1043, event data cluster=TRUE ("event data")) -> ()  [unwired: 2 in, 2 out]
          }
        }
      }
      frame "Calibrate Force" {
        n507 = in-place {
          in-place-border: [w1184] -> w1139
          in-place-border: [w1183] -> w1133
          in-place-border: [w1182] -> w1117
          n508 = in-place-cluster #38(w1140) -> ("Task Ref"=w1186:refnum<vi>, "Shut Down"=w1183:refnum<user-event>, "Calibrate Force"=w1182:refnum<user-event>)
          n509 = property class="DAQmxName (strict)"(reference=w1186) -> (reference out=w1185:refnum<vi>, "Value"=w1184:refnum<k21>)  [unwired: 1 in, 1 out]
          n510 = in-place-cluster #38("Task Ref"=w1185, "Shut Down"=w1183, "Calibrate Force"=w1182) -> (w1121:refnum<class "NI Force Task.lvclass">)
        }
        n511 = Obtain Queue(name (unnamed)="Calibration Q", element data type=waveform(dbl)[] [] ("data")) -> (queue out=w1134:refnum<queue>, error out=w1128:errorcluster)  [unwired: 3 in, 1 out]
        n512 = call <vilib>:"DAQmx Start Task.vi"("task/channels in"=w1139) -> ("task out"=w1138:refnum<k21>, "error out"=w1137:errorcluster)  [unwired: 13 in]
        n513 = while {
          tunnel: w1134 -> [w1150]
          tunnel: w1128 -> [w1149]
          tunnel: [w1147] -> w1127
          tunnel: [w1146] -> w1126
          tunnel: [w1142] -> w1125 mode=concatenating
          tunnel: [w1141] -> w1124 mode=concatenating
          stop <- w1148 stop-if-true
          n514 = Dequeue Element(queue=w1150, error in (no error)=w1149) -> (queue out=w1147:refnum<queue>, element=w1143:waveform(dbl)[], error out=w1146:errorcluster)  [unwired: 1 in, 1 out]
          n515 = in-place {
            in-place-border: [w1152] -> w1142
            in-place-border: [w1151] -> w1141
            n516 = in-place-array #39(w1143, 0, 1) -> (w1156:waveform(dbl), w1155:waveform(dbl))
            n517 = in-place {
              in-place-border: [w1158] -> w1152
              in-place-border: [w1157] -> w1151
              n518 = in-place-cluster #40(w1156) -> ("Y"=w1158:dbl[])
              n519 = in-place-cluster #41(w1155) -> ("Y"=w1157:dbl[])
              n520 = in-place-cluster #40("Y"=w1158) -> (w1154:waveform(dbl))
              n521 = in-place-cluster #41("Y"=w1157) -> (w1153:waveform(dbl))
            }
            n522 = in-place-array #39(w1154, w1153) -> ()  [unwired: 3 out]
          }
          n523 = Empty Array?(array=w1143) -> (empty?=w1148:bool)
        }
        n524 = while {
          tunnel: w1138 -> [w1170]
          tunnel: w1137 -> [w1169]
          tunnel: w1134 -> [w1168]
          tunnel: w1133 -> [w1165]
          tunnel: [w1164] -> w1132
          tunnel: [w1160] -> w1131
          tunnel: [w1159] -> w1130
          stop <- w1163 stop-if-true
          n525 = call-poly <vilib>:"DAQmx Read.vi"("task/channels in"=w1170, "error in"=w1169) -> ("task out"=w1164:refnum<k21>, "data"=w1166:waveform(dbl)[], "error out"=w1167:errorcluster)  [unwired: 11 in]
          n526 = case shown="No Error" w1167 {
            selector: w1167 -> [_ w1179]
            tunnel: w1168 -> [w1175 w1181]
            tunnel: w1166 -> [w1174 _]
            tunnel: [w1173 w1181] -> w1160
            tunnel: [FALSE ("x") w1180] -> w1161
            tunnel: w1165 -> [_ w1177]
            tunnel: [w1171 errorcluster {"status"=FALSE, "code"=0, "source"=""} ("error out")] -> w1159
            frame No Error {
              n527 = Enqueue Element(queue=w1175, element=w1174) -> (queue out=w1173:refnum<queue>, error out=w1171:errorcluster)  [unwired: 2 in, 1 out]
            }
            frame Error {
              n528 = Generate User Event(user event=w1177, event data cluster=TRUE ("event data")) -> ()  [unwired: 2 in, 2 out]
              n529 = Unbundle By Name(w1179) -> ("status"=w1180:bool)
            }
          }
          n530 = property on="Stop Acquire" class="Bool (strict)"() -> ("Value"=w1162:bool)  [unwired: 2 in, 2 out]
          n531 = Or(x=w1161, y=w1162) -> (x .or. y?=w1163:bool)
        }
        n532 = Release Queue(queue=w1127, error in (no error)=w1126) -> ()  [unwired: 1 in, 3 out]
        n533 = call-poly <vilib>:"Mean.vi"("X"=w1124) -> ("mean"=w1123:dbl)  [unwired: 1 out]
        n534 = call-poly <vilib>:"Mean.vi"("X"=w1125) -> ("mean"=w1122:dbl)  [unwired: 1 out]
        n535 = Bundle("mean"=w1122, "mean"=w1123) -> (w1119:cluster{"mean":dbl, "mean":dbl})  [unwired: 1 in]
        n536 = call <vilib>:"Read Caller Enqueuer.vi"("Actor"=w1121) -> ("Caller Enqueuer"=w1120:refnum<class "Message Enqueuer.lvclass">)  [unwired: 10 in]
        n537 = Enqueue Element(queue=w1131, element=waveform(dbl)[] [] ("data"), error in (no error)=w1130) -> ()  [unwired: 1 in, 3 out]
        n538 = call <vilib>:"DAQmx Stop Task.vi"("task/channels in"=w1132) -> ()  [unwired: 13 in, 2 out]
        n539 = call "Send Force Calibration Finished.vi"("Force calibratred values"=w1119, "Message Enqueuer"=w1120) -> ("error out"=w1118:errorcluster)  [unwired: 8 in, 1 out]
        n540 = Generate User Event(user event=w1117, event data cluster=FALSE ("event data"), error in=w1118) -> ()  [unwired: 1 in, 2 out]
      }
      frame "Calibrate Potentiometers" {
        n541 = in-place {
          in-place-border: [w1255] -> w1210
          in-place-border: [w1254] -> w1204
          in-place-border: [w1253] -> w1188
          n542 = in-place-cluster #42(w1211) -> ("Task Ref"=w1257:refnum<vi>, "Shut Down"=w1254:refnum<user-event>, "Calibrate Pot"=w1253:refnum<user-event>)
          n543 = property class="DAQmxName (strict)"(reference=w1257) -> (reference out=w1256:refnum<vi>, "Value"=w1255:refnum<k21>)  [unwired: 1 in, 1 out]
          n544 = in-place-cluster #42("Task Ref"=w1256, "Shut Down"=w1254, "Calibrate Pot"=w1253) -> (w1192:refnum<class "NI Force Task.lvclass">)
        }
        n545 = Obtain Queue(name (unnamed)="Calibration Q", element data type=waveform(dbl)[] [] ("data")) -> (queue out=w1205:refnum<queue>, error out=w1199:errorcluster)  [unwired: 3 in, 1 out]
        n546 = call <vilib>:"DAQmx Start Task.vi"("task/channels in"=w1210) -> ("task out"=w1209:refnum<k21>, "error out"=w1208:errorcluster)  [unwired: 13 in]
        n547 = while {
          tunnel: w1205 -> [w1221]
          tunnel: w1199 -> [w1220]
          tunnel: [w1218] -> w1198
          tunnel: [w1217] -> w1197
          tunnel: [w1213] -> w1196 mode=concatenating
          tunnel: [w1212] -> w1195 mode=concatenating
          stop <- w1219 stop-if-true
          n548 = Dequeue Element(queue=w1221, error in (no error)=w1220) -> (queue out=w1218:refnum<queue>, element=w1214:waveform(dbl)[], error out=w1217:errorcluster)  [unwired: 1 in, 1 out]
          n549 = in-place {
            in-place-border: [w1223] -> w1213
            in-place-border: [w1222] -> w1212
            n550 = in-place-array #43(w1214, 0, 1) -> (w1227:waveform(dbl), w1226:waveform(dbl))
            n551 = in-place {
              in-place-border: [w1229] -> w1223
              in-place-border: [w1228] -> w1222
              n552 = in-place-cluster #44(w1227) -> ("Y"=w1229:dbl[])
              n553 = in-place-cluster #45(w1226) -> ("Y"=w1228:dbl[])
              n554 = in-place-cluster #44("Y"=w1229) -> (w1225:waveform(dbl))
              n555 = in-place-cluster #45("Y"=w1228) -> (w1224:waveform(dbl))
            }
            n556 = in-place-array #43(w1225, w1224) -> ()  [unwired: 3 out]
          }
          n557 = Empty Array?(array=w1214) -> (empty?=w1219:bool)
        }
        n558 = while {
          tunnel: w1209 -> [w1241]
          tunnel: w1208 -> [w1240]
          tunnel: w1205 -> [w1239]
          tunnel: w1204 -> [w1236]
          tunnel: [w1235] -> w1203
          tunnel: [w1231] -> w1202
          tunnel: [w1230] -> w1201
          stop <- w1234 stop-if-true
          n559 = call-poly <vilib>:"DAQmx Read.vi"("task/channels in"=w1241, "error in"=w1240) -> ("task out"=w1235:refnum<k21>, "data"=w1237:waveform(dbl)[], "error out"=w1238:errorcluster)  [unwired: 11 in]
          n560 = case shown="No Error" w1238 {
            selector: w1238 -> [_ w1250]
            tunnel: w1239 -> [w1246 w1252]
            tunnel: w1237 -> [w1245 _]
            tunnel: [w1244 w1252] -> w1231
            tunnel: [FALSE ("x") w1251] -> w1232
            tunnel: w1236 -> [_ w1248]
            tunnel: [w1242 errorcluster {"status"=FALSE, "code"=0, "source"=""} ("error out")] -> w1230
            frame No Error {
              n561 = Enqueue Element(queue=w1246, element=w1245) -> (queue out=w1244:refnum<queue>, error out=w1242:errorcluster)  [unwired: 2 in, 1 out]
            }
            frame Error {
              n562 = Generate User Event(user event=w1248, event data cluster=TRUE ("event data")) -> ()  [unwired: 2 in, 2 out]
              n563 = Unbundle By Name(w1250) -> ("status"=w1251:bool)
            }
          }
          n564 = property on="Stop Acquire" class="Bool (strict)"() -> ("Value"=w1233:bool)  [unwired: 2 in, 2 out]
          n565 = Or(x=w1232, y=w1233) -> (x .or. y?=w1234:bool)
        }
        n566 = Release Queue(queue=w1198, error in (no error)=w1197) -> ()  [unwired: 1 in, 3 out]
        n567 = call-poly <vilib>:"Mean.vi"("X"=w1195) -> ("mean"=w1194:dbl)  [unwired: 1 out]
        n568 = call-poly <vilib>:"Mean.vi"("X"=w1196) -> ("mean"=w1193:dbl)  [unwired: 1 out]
        n569 = Bundle("mean"=w1193, "mean"=w1194) -> (w1190:cluster{"mean":dbl, "mean":dbl})  [unwired: 1 in]
        n570 = call <vilib>:"Read Caller Enqueuer.vi"("Actor"=w1192) -> ("Caller Enqueuer"=w1191:refnum<class "Message Enqueuer.lvclass">)  [unwired: 10 in]
        n571 = Enqueue Element(queue=w1202, element=waveform(dbl)[] [] ("data"), error in (no error)=w1201) -> ()  [unwired: 1 in, 3 out]
        n572 = call <vilib>:"DAQmx Stop Task.vi"("task/channels in"=w1203) -> ()  [unwired: 13 in, 2 out]
        n573 = call "Send Pot Calibration Finished.vi"("Pot calibratred values"=w1190, "Message Enqueuer"=w1191) -> ("error out"=w1189:errorcluster)  [unwired: 8 in, 1 out]
        n574 = Generate User Event(user event=w1188, event data cluster=FALSE ("event data"), error in=w1189) -> ()  [unwired: 1 in, 2 out]
      }
    }
  }
  n575 = call-parent "Actor Core.vi"("error in"=w15, "Panel Actor in"=w4) -> ("error out"=→"error out":errorcluster, "Actor out"=→"Actor out":refnum<class "Actor.lvclass">)  [unwired: 8 in]
  n576 = Unregister For Events(event registration refnum=w9) -> ()  [unwired: 1 in, 1 out]
